vi "Sequence.vi"(8 "error in (no error)":errorcluster, 11 "Message Queues in":T73) -> (0 "error out":errorcluster)   [LabVIEW 2018, in "Sequencing Library.lvlib"]
uses:
  Sequencing Library.lvlib
  Main/Main Queue Cluster.ctl
  support/Message Queue/Message Cluster.ctl
  Drag and Drop/State Cluster.ctl
  Drag and Drop/Thumbnail Cluster.ctl
  Drag and Drop/Object Cluster.ctl
  <vilib>/Utility/miscctls.llb/LVRectTypeDef.ctl
  Drag and Drop/Object Type Enum.ctl
  <vilib>/Utility/miscctls.llb/LVPositionTypeDef.ctl
  Config Module/Controls/Main Config Cluster.ctl
  OPC/OPC Module Config.ctl
  Scale Module Folder/Measure Instrument/State Enum.ctl
  <vilib>/Utility/miscctls.llb/LVPoint32TypeDef.ctl
  OPC/OPC Settings.ctl
  OPC/Variable Data Cluster.ctl
  <vilib>/OPCUA/controls/NodeId.ctl
  <vilib>/OPCUA/controls/OPC UA StatusCode.ctl
  <vilib>/OPCUA/controls/Subscription ID.ctl
  <vilib>/OPCUA/controls/OPC UA Client Refnum.ctl
  <vilib>/OPCUA/controls/Subscription Data Change.ctl
  <vilib>/OPCUA/controls/Data Type.ctl
  OPC/OPC Tag Data.ctl
  Feed Module/Controls/Feed Module Config Cluster.ctl
  Feed Module/Controls/Feed Module Settings Cluster.ctl
  Ismatec ISM 831C/Controls/Ismatech ISM831C Settings Cluster.ctl
  Masterflex 7550-30/Controls/Settings Cluster.ctl
  Mettler Toledo/Controls/Settings Cluster.ctl
  Bronkhorst M13 Flow Meter/Settings Cluster.ctl
  Measure Instrument/PID 2 Parameters Cluster.ctl
  Measure Instrument/PID Input Enum.ctl
  Measure Instrument/PID 2 Output Enum.ctl
  Tacmina QI/Tacmina QI DAQ Setting.ctl
  KNF Pump/Settings Cluster plus SIMDOS.ctl
  ASIA Pump/Pump Settings.ctl
  VICI M50 Party Mode/Settings Cluster.ctl
  FLOM Pump/Settings Cluster.ctl
  SSI PR Class/SSI PR or LD Settings Cluster.ctl
  Masterflex 75211/Masterflex 75211 DAQ Setting.ctl
  SSI PR Class/SSI P40 Settings Cluster.ctl
  Ismatec 78001/Ismatec 4083.ctl
  Bronkhorst M14 Flow Meter/Settings Cluster.ctl
  TT Module/Controls/TT Module Config Cluster.ctl
  Tag VIs/Numeric Alarm Settings Cluster.ctl
  Acquisition/Hardware Configuration.ctl
  Acquisition/Task Cluster.ctl
  PT Module/Controls/PT Module Config Cluster.ctl
  Scale Module Folder/Feed Module/Controls/Scale Module Config Cluster.ctl
  Scale Module Folder/Feed Module/Controls/Scale Module Settings Cluster.ctl
  Pump Module Folder/Pump Module Config Cluster.ctl
  Pump Module Folder/Pump Module Settings Cluster.ctl
  LabJack Module/Controls/U3 Module Config Cluster.ctl
  Decoration Module/Decoration Module Config Cluster.ctl
  Flow Module Folder/Feed Module/Controls/Flow Module Config Cluster.ctl
  Flow Module Folder/Feed Module/Controls/Flow Module Settings Cluster.ctl
  TCU Module/TCU Module Folder/TCU Module Config Cluster.ctl
  TCU Module/TCU Module Folder/TCU Module Settings Cluster.ctl
  TCU Module/TCU Module Folder/Measure Instrument/Output Devices.ctl
  Huber TCU/Huber Settings.ctl
  Lauda Integral XT-150 TCU/Lauda Settings.ctl
  Julabo Type 1 TCU/Julabo Type 1 TCU Folder/Julabo FP-50 Settings.ctl
  Huber Unistat 410 TCU/Huber Unistat 410 RS485 Settings.ctl
  D-O Module Folder/Not Sure Where this is Used.ctl
  Squence Control.ctl
  D-O Module Folder/D-O Module Config Cluster.ctl
  D-O Module Folder/Valve Clusters.ctl
  D-O Module Folder/D-O Module Settings Cluster.ctl
  D-O Module Folder/D-O Device Settings Cluster.ctl
  VICI Electronic Actuator/VICI Electronic Actuator Settings.ctl
  Pressure Regulator Control Module/Pressure Regulator/Controls/4-20mA Module Config Cluster.ctl
  Pressure Regulator Control Module/Pressure Regulator/Controls/4-20mA Module Settings Cluster.ctl
  Pressure Transmitter/Pressure Transmitter Device Settings.ctl
  Pressure Reg Module/Pressure Regulator Device Settings.ctl
  Sonicator Module Folder/Feed Module/Controls/Sonicator Module Config Cluster.ctl
  Sonicator Module Folder/Feed Module/Controls/Sonicator Module Settings Cluster.ctl
  Sonic Systems P100/Sonic Systems P100 Settings.ctl
  Agitator Module Folder/Feed Module/Controls/Agitator Module Config Cluster.ctl
  Agitator Module Folder/Feed Module/Controls/Agitator Module Settings Cluster.ctl
  Squence Update Cluster.ctl
  support/Message Queue/Enqueue Message (Single).vi
  support/Message Queue/Message Queue.lvlib
  support/Command Log VIs/Command Logging.lvlib
  Drag and Drop/Drag and Drop.lvlib
  Config Module/Config Module.lvlib
  TT Module/TT Module.lvlib
  Feed Module/Feed Module.lvlib
  Ismatec ISM 831C/Ismatec ISM 831C.lvlib
  Masterflex 7550-30/Masterflex 7550-30.lvlib
  Mettler Toledo/Mettler Toledo.lvlib
  Bronkhorst M13 Flow Meter/Bronkhorst M13 Flow Meter.lvlib
  Tacmina QI/Tacmina QI.lvlib
  KNF Pump/KNF SIMDOS.lvlib
  ASIA Pump.lvlib
  DAQ/DAQ.lvlib
  PT Module/PT Module.lvlib
  Scale Module Folder/Scale Module.lvlib
  Pump Module Folder/Pump Module.lvlib
  LabJack Module/U3 Module.lvlib
  Flow Module Folder/Flow Module.lvlib
  TCU Module/TCU Module Folder/TCU Module.lvlib
  Huber TCU/Huber Ministat 230 TCU.lvlib
  Lauda Integral XT-150 TCU/Lauda TCU.lvlib
  Julabo Type 1 TCU/Julabo Type 1 TCU Folder/Julabo Type FP-50 TCU.lvlib
  VICI M50 Party Mode/VICI M6 M50 Party Mode.lvlib
  D-O Module Folder/D-O Module.lvlib
  Pressure Transmitter/Pressure Transmitter Library.lvlib
  Pressure Regulator Control Module/Pressure Regulator/4-20mA Module.lvlib
  Pressure Reg Module/Pressure Regulator Library.lvlib
  FLOM Pump/FLOM Pump.lvlib
  SSI PR Class/SSI PR or LD Pump.lvlib
  OPC/OPC UA.lvlib
  Scale Module Folder/Measure Instrument/Scale Module Engine.lvlib
  D-O Module Folder/DIO Valve/VICI Electronic Actuator.lvlib
  Masterflex 75211/Masterflex 75211.lvlib
  SSI PR Class/SSI P40 Pump.lvlib
  Huber Unistat 410 TCU/Huber Unistat 410 TCU.lvlib
  Ismatec 78001/Ismatec 4308.lvlib
  Bronkhorst M14 Flow Meter/Bronkhorst M14 Flow Meter.lvlib
  Sonicator Module Folder/Sonicator Module.lvlib
  Sonic Systems P100/Sonic Systems P100.lvlib
  Agitator Module Folder/Agitator Module.lvlib
panel:
  in  "Input 2":T1 {"Main Config"."PR Module Configs"."Settings"."PID 2 Parameters"."output range"."output low" format="%.2f"; "Main Config"."PR Module Configs"."Settings"."PID 2 Parameters"."output range"."output high" min=0.0 max=100.0 format="%.2f"; "Main Config"."PR Module Configs"."Settings"."PID 2 Parameters"."PID gains"."derivative time (Td, min)" format="%.3f"; "Main Config"."PR Module Configs"."Settings"."PID 2 Parameters"."PID gains"."integral time (Ti, min)" format="%.3f"; "Main Config"."PR Module Configs"."Settings"."PID 2 Parameters"."PID gains"."proportional gain (Kc)" format="%.3f"; "Main Config"."Steps"."Control" items=["Pump %", "Setpoint"]; "Main Config"."TCU Module Configs"."Settings"."Huber Unistat 410 Settings"."Address" min=0 max=99 format="%02.0f"; "Main Config"."TCU Module Configs"."Settings"."Julabo FP-50 Settings"."Pump Power" min=0 max=8 step=1; "Main Config"."TCU Module Configs"."Settings"."Lauda Settings"."Pump Power" min=0 max=8 step=1; "Main Config"."Flow Module Configs"."Settings"."Bronkhorst M14 Settings"."Smoothing Steps" min=1 step=1; "Main Config"."Flow Module Configs"."Settings"."Bronkhorst M13 Settings"."Smoothing Steps" min=1 step=1; "Main Config"."Pump Module Configs"."Settings"."Ismatech 3 Channel Settings"."Channel Number" min=0 max=3; "Main Config"."Pump Module Configs"."Settings"."Ismatech 3 Channel Settings"."Pump Number" min=1; "Main Config"."Pump Module Configs"."Settings"."ASIA Pump C"."channel" min=0 max=1 step=1; "Main Config"."Pump Module Configs"."Settings"."Masterflex"."Pump Number" min=1.0 max=20.0 step=1.0; "Main Config"."Pump Module Configs"."Settings"."Ismatech"."Pump Number" min=1.0 max=20.0 step=1.0; "Main Config"."Feed Module Configs"."Settings"."Bronkhorst M14 Settings"."Smoothing Steps" min=1 step=1; "Main Config"."Feed Module Configs"."Settings"."Ismatech 3 Channel Settings"."Channel Number" min=0 max=3; "Main Config"."Feed Module Configs"."Settings"."Ismatech 3 Channel Settings"."Pump Number" min=1; "Main Config"."Feed Module Configs"."Settings"."output range"."output low" min=0.0 max=100.0 format="%.2f"; "Main Config"."Feed Module Configs"."Settings"."output range"."output high" format="%.2f"; "Main Config"."Feed Module Configs"."Settings"."PID 2 Parameters"."PID gains"."derivative time (Td, min)" format="%.3f"; "Main Config"."Feed Module Configs"."Settings"."PID 2 Parameters"."PID gains"."integral time (Ti, min)" format="%.3f"; "Main Config"."Feed Module Configs"."Settings"."PID 2 Parameters"."PID gains"."proportional gain (Kc)" format="%.3f"; "Main Config"."Feed Module Configs"."Settings"."Bronkhorst M13 Flow Meter"."Smoothing Steps" min=1 step=1; "Main Config"."Feed Module Configs"."Settings"."ASIA Pump C"."channel" min=0 max=1 step=1; "Main Config"."Feed Module Configs"."Settings"."Ismatech"."Pump Number" min=1.0 max=20.0 step=1.0; "Main Config"."Feed Module Configs"."Settings"."Masterflex"."Pump Number" min=1.0 max=20.0 step=1.0}
  out "Metrics:Code Size":u32
  out "Metrics:Total Data Size":u32
  out "Application:All VIs In Memory":string[](array[string])
  out "error out 2":errorcluster
  out "Process Name":string
  out "Queue Name":string
  out "Loop Variable":u32
  out "Step":i32
  out "Done":bool
  out "Output":T1 {"Main Config"."PR Module Configs"."Settings"."PID 2 Parameters"."output range"."output low" format="%.2f"; "Main Config"."PR Module Configs"."Settings"."PID 2 Parameters"."output range"."output high" min=0.0 max=100.0 format="%.2f"; "Main Config"."PR Module Configs"."Settings"."PID 2 Parameters"."PID gains"."derivative time (Td, min)" format="%.3f"; "Main Config"."PR Module Configs"."Settings"."PID 2 Parameters"."PID gains"."integral time (Ti, min)" format="%.3f"; "Main Config"."PR Module Configs"."Settings"."PID 2 Parameters"."PID gains"."proportional gain (Kc)" format="%.3f"; "Main Config"."Steps"."Control" items=["Pump %", "Setpoint"]; "Main Config"."TCU Module Configs"."Settings"."Huber Unistat 410 Settings"."Address" min=0 max=99 format="%02.0f"; "Main Config"."TCU Module Configs"."Settings"."Julabo FP-50 Settings"."Pump Power" min=0 max=8 step=1; "Main Config"."TCU Module Configs"."Settings"."Lauda Settings"."Pump Power" min=0 max=8 step=1; "Main Config"."Flow Module Configs"."Settings"."Bronkhorst M14 Settings"."Smoothing Steps" min=1 step=1; "Main Config"."Flow Module Configs"."Settings"."Bronkhorst M13 Settings"."Smoothing Steps" min=1 step=1; "Main Config"."Pump Module Configs"."Settings"."Ismatech 3 Channel Settings"."Channel Number" min=0 max=3; "Main Config"."Pump Module Configs"."Settings"."Ismatech 3 Channel Settings"."Pump Number" min=1; "Main Config"."Pump Module Configs"."Settings"."ASIA Pump C"."channel" min=0 max=1 step=1; "Main Config"."Pump Module Configs"."Settings"."Masterflex"."Pump Number" min=1.0 max=20.0 step=1.0; "Main Config"."Pump Module Configs"."Settings"."Ismatech"."Pump Number" min=1.0 max=20.0 step=1.0; "Main Config"."Feed Module Configs"."Settings"."Bronkhorst M14 Settings"."Smoothing Steps" min=1 step=1; "Main Config"."Feed Module Configs"."Settings"."Ismatech 3 Channel Settings"."Channel Number" min=0 max=3; "Main Config"."Feed Module Configs"."Settings"."Ismatech 3 Channel Settings"."Pump Number" min=1; "Main Config"."Feed Module Configs"."Settings"."output range"."output low" min=0.0 max=100.0 format="%.2f"; "Main Config"."Feed Module Configs"."Settings"."output range"."output high" format="%.2f"; "Main Config"."Feed Module Configs"."Settings"."PID 2 Parameters"."PID gains"."derivative time (Td, min)" format="%.3f"; "Main Config"."Feed Module Configs"."Settings"."PID 2 Parameters"."PID gains"."integral time (Ti, min)" format="%.3f"; "Main Config"."Feed Module Configs"."Settings"."PID 2 Parameters"."PID gains"."proportional gain (Kc)" format="%.3f"; "Main Config"."Feed Module Configs"."Settings"."Bronkhorst M13 Flow Meter"."Smoothing Steps" min=1 step=1; "Main Config"."Feed Module Configs"."Settings"."ASIA Pump C"."channel" min=0 max=1 step=1; "Main Config"."Feed Module Configs"."Settings"."Ismatech"."Pump Number" min=1.0 max=20.0 step=1.0; "Main Config"."Feed Module Configs"."Settings"."Masterflex"."Pump Number" min=1.0 max=20.0 step=1.0}
  out "Intruction Cluster":T58 {"Control" items=["Setpoint", "Pump %"]}
  out "Paused":bool
  out "Stop":bool
  in  "Input":T1 {"Main Config"."PR Module Configs"."Settings"."PID 2 Parameters"."output range"."output low" format="%.2f"; "Main Config"."PR Module Configs"."Settings"."PID 2 Parameters"."output range"."output high" min=0.0 max=100.0 format="%.2f"; "Main Config"."PR Module Configs"."Settings"."PID 2 Parameters"."PID gains"."derivative time (Td, min)" format="%.3f"; "Main Config"."PR Module Configs"."Settings"."PID 2 Parameters"."PID gains"."integral time (Ti, min)" format="%.3f"; "Main Config"."PR Module Configs"."Settings"."PID 2 Parameters"."PID gains"."proportional gain (Kc)" format="%.3f"; "Main Config"."Steps"."Control" items=["Pump %", "Setpoint"]; "Main Config"."TCU Module Configs"."Settings"."Huber Unistat 410 Settings"."Address" min=0 max=99 format="%02.0f"; "Main Config"."TCU Module Configs"."Settings"."Julabo FP-50 Settings"."Pump Power" min=0 max=8 step=1; "Main Config"."TCU Module Configs"."Settings"."Lauda Settings"."Pump Power" min=0 max=8 step=1; "Main Config"."Flow Module Configs"."Settings"."Bronkhorst M14 Settings"."Smoothing Steps" min=1 step=1; "Main Config"."Flow Module Configs"."Settings"."Bronkhorst M13 Settings"."Smoothing Steps" min=1 step=1; "Main Config"."Pump Module Configs"."Settings"."Ismatech 3 Channel Settings"."Channel Number" min=0 max=3; "Main Config"."Pump Module Configs"."Settings"."Ismatech 3 Channel Settings"."Pump Number" min=1; "Main Config"."Pump Module Configs"."Settings"."ASIA Pump C"."channel" min=0 max=1 step=1; "Main Config"."Pump Module Configs"."Settings"."Masterflex"."Pump Number" min=1.0 max=20.0 step=1.0; "Main Config"."Pump Module Configs"."Settings"."Ismatech"."Pump Number" min=1.0 max=20.0 step=1.0; "Main Config"."Feed Module Configs"."Settings"."Bronkhorst M14 Settings"."Smoothing Steps" min=1 step=1; "Main Config"."Feed Module Configs"."Settings"."Ismatech 3 Channel Settings"."Channel Number" min=0 max=3; "Main Config"."Feed Module Configs"."Settings"."Ismatech 3 Channel Settings"."Pump Number" min=1; "Main Config"."Feed Module Configs"."Settings"."output range"."output low" min=0.0 max=100.0 format="%.2f"; "Main Config"."Feed Module Configs"."Settings"."output range"."output high" format="%.2f"; "Main Config"."Feed Module Configs"."Settings"."PID 2 Parameters"."PID gains"."derivative time (Td, min)" format="%.3f"; "Main Config"."Feed Module Configs"."Settings"."PID 2 Parameters"."PID gains"."integral time (Ti, min)" format="%.3f"; "Main Config"."Feed Module Configs"."Settings"."PID 2 Parameters"."PID gains"."proportional gain (Kc)" format="%.3f"; "Main Config"."Feed Module Configs"."Settings"."Bronkhorst M13 Flow Meter"."Smoothing Steps" min=1 step=1; "Main Config"."Feed Module Configs"."Settings"."ASIA Pump C"."channel" min=0 max=1 step=1; "Main Config"."Feed Module Configs"."Settings"."Ismatech"."Pump Number" min=1.0 max=20.0 step=1.0; "Main Config"."Feed Module Configs"."Settings"."Masterflex"."Pump Number" min=1.0 max=20.0 step=1.0}
  # "Agitator Settings"
  # "Sonicator Settings"
  # "Instrument Settings"
  # "Instrument Settings"
  # "Output Instruments"
  # "Flow Meter Settings"
  # "Output Instruments"
  # "Scale Settings"
  # "Output Instruments"
  # "Input Instruments"
  # "Agitator Settings"
  # "Sonicator Settings"
  # "Instrument Settings"
  # "Instrument Settings"
  # "Output Instruments"
  # "Flow Meter Settings"
  # "Output Instruments"
  # "Scale Settings"
  # "Output Instruments"
  # "Input Instruments"
  # "Agitator Settings"
  # "Sonicator Settings"
  # "Instrument Settings"
  # "Instrument Settings"
  # "Output Instruments"
  # "Flow Meter Settings"
  # "Output Instruments"
  # "Scale Settings"
  # "Output Instruments"
  # "Input Instruments"
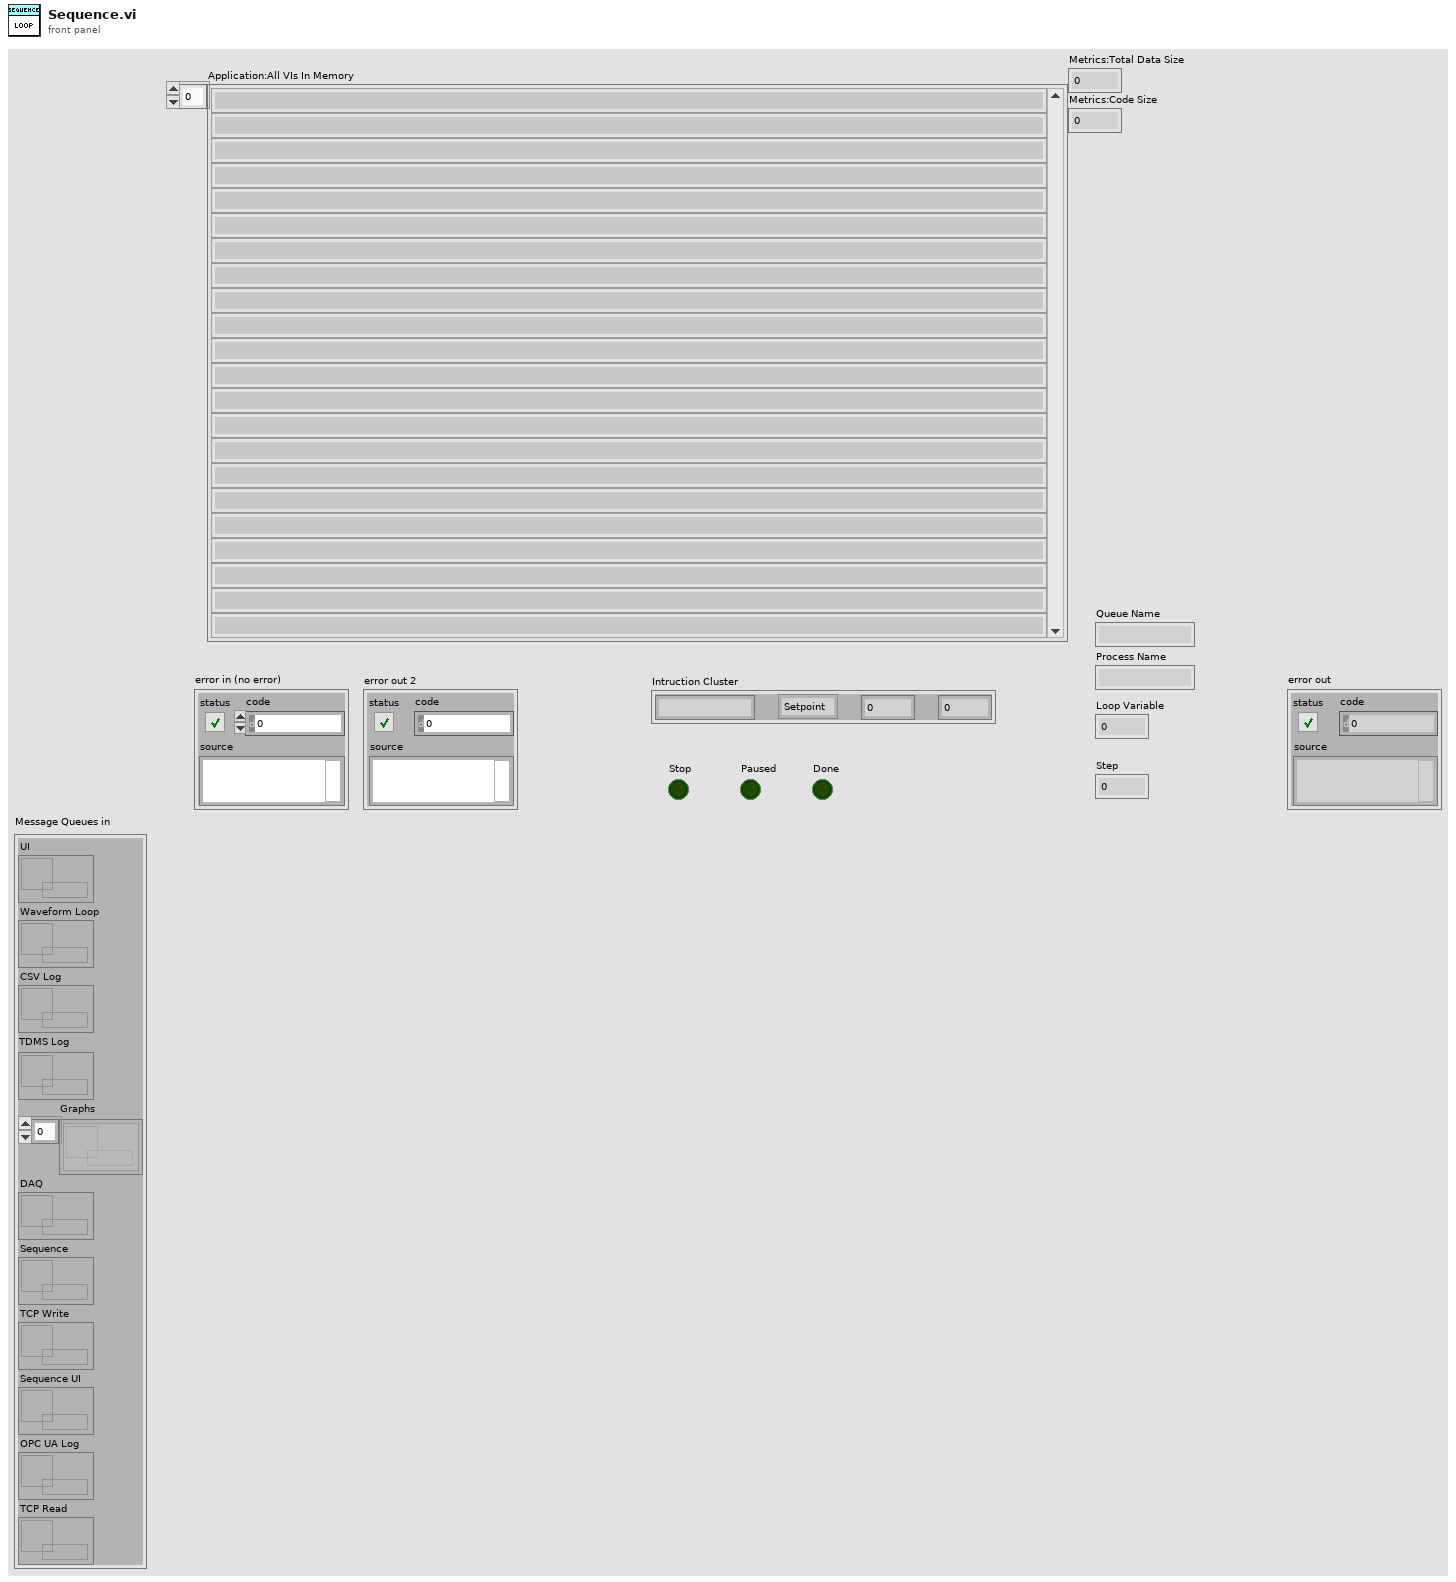
[diagram p1: front panel]
types:
  T1 = typedef "Drag and Drop.lvlib/State Cluster.ctl" = cluster{"VI refs":refnum<vi>[], "Queues":refnum<queue>[], "[Thumbnails]":T2[], "Drag Object Idx":i32, "[Objects]":T3[], "Active Object":i32, "Drop Offset":T6, "Process Name":string, "Main Config":T7, "Campaign Filepath":path, "Config Changed?":bool}
  T2 = typedef "Thumbnail Cluster.ctl" = cluster{"Path":path, "Rectangle":cluster{"left":i16, "top":i16, "right":i16, "bottom":i16}}
  T3 = typedef "Object Cluster.ctl" = cluster{"BMP Path":path, "Anchor Position":cluster{"X":i32, "Y":i32}, "Hot Spot":T4, "Type":T5, "Parameters":variant}
  T4 = typedef "LVRectTypeDef.ctl" = cluster{"Left":i16, "Top":i16, "Right":i16, "Bottom":i16}
  T5 = typedef "Object Type Enum.ctl" = enum16{"Icon", "Line", "Text", "Feed Module"}
  T6 = typedef "LVPositionTypeDef.ctl" = cluster{"Left":i32, "Top":i32}
  T7 = typedef "Config Module.lvlib/Main Config Cluster.ctl" = cluster{"Notebook":string, "OPC Module Configs":T8[], "Feed Module Configs":T18[], "Log File Path":path, "TT Module Configs":T37[], "DAQ Config":T39, "PT Module Configs":T41[], "Scale Module Configs":T42[], "Pump Module Configs":T44[], "U3 Module Configs":T46[], "Decoration Module Configs":T47[], "Flow Module Configs":T48[], "TCU Module Configs":T50[], "Steps":T57, "Abort":bool, "DO Module Configs":T59[], "PR Module Configs":T64[], "SC Module Configs":T68[], "AM Module Configs":T71[], "Cycle Period":dbl}
  T8 = typedef "OPC UA.lvlib/OPC Module Config.ctl" = cluster{"State":T9, "GUID":string, "Drop Coords":T10, "Configuration":T11, "First Iteration":bool, "Data":cluster{"Object Name":string, "Variable Array":T12[]}[], "Process Name":string, "Load Count":i32, "Log Started":bool, "subscription ID out":T15, "OPC UA client refnum out":T16, "Event Registration Refnum":refnum<event-registration>, "Start Time":timestamp, "Current Time":timestamp, "Tag Data":T17[]}
  T9 = typedef "Scale Module.lvlib/Scale Module Engine.lvlib/State Enum.ctl" = enum16{"Measuring", "Idle"}
  T10 = typedef "LVPoint32TypeDef.ctl" = cluster{"Horizontal":i32, "Vertical":i32}
  T11 = typedef "OPC UA.lvlib/OPC Settings.ctl" = cluster{"Cycle Period":dbl, "server endpoint URL":string, "security policy":cluster{"message mode":enum16{"None", "Sign", "Sign and Encrypt"}, "security":enum16{"Basic256", "Basic128Rsa15"}}, "Trust Any Server":bool}
  T12 = typedef "OPC UA.lvlib/Variable Data Cluster.ctl" = cluster{"node ID":T13, "browse name":string, "status":T14, "timestamp":timestamp, "value ":variant}
  T13 = typedef "NodeId.ctl" = string
  T14 = typedef "OPC UA StatusCode.ctl" = u32
  T15 = typedef "Subscription ID.ctl" = u32
  T16 = typedef "OPC UA Client Refnum.ctl" = refnum<k21>
  T17 = typedef "OPC UA.lvlib/OPC Tag Data.ctl" = cluster{"Include this Device":bool, "Device Name":string, "OPC Tag Data":cluster{"Tag":string, "Value":variant, "Time Stamp":timestamp}[]}
  T18 = typedef "Feed Module.lvlib/Feed Module Config Cluster.ctl" = cluster{"GUID":string, "Drop Coords":T10, "Process Name":string, "Queue Name":string, "Settings":T19, "Settings Load Count":i32, "OP Load Count":i32}
  T19 = typedef "Feed Module.lvlib/Feed Module Settings Cluster.ctl" = cluster{"Cycle Period":dbl, "Ismatech":T20, "Masterflex":T21, "Mettler":T22, "Bronkhorst M13 Flow Meter":T23, "PID 2 Parameters":T24, "Manual Entry":dbl, "Auto?":bool, "output range":cluster{"output high":dbl, "output low":dbl}, "Tacmina Settings":T27, "KNF SIMDOS Settings":T28, "ASIA Pump C":T29, "VICI Settings":T30, "FLOM Settings":T31, "SSI PR/LD Settings":T32, "Masterflex 75211 Settings":T33, "SSI P40 Settings":T34, "Ismatech 3 Channel Settings":T35, "Bronkhorst M14 Settings":T36}
  T20 = typedef "Ismatec ISM 831C.lvlib/Ismatech ISM831C Settings Cluster.ctl" = cluster{"VISA resource name":refnum<visa-resource-name>, "Simulated?":bool, "Pump Number":dbl, "Reverse?":bool}
  T21 = typedef "Masterflex 7550-30.lvlib/Settings Cluster.ctl" = cluster{"VISA resource name":refnum<visa-resource-name>, "Simulated?":bool, "Pump Number":dbl, "Reverse?":bool}
  T22 = typedef "Mettler Toledo.lvlib/Settings Cluster.ctl" = cluster{"VISA resource name":refnum<visa-resource-name>, "Simulated?":bool}
  T23 = typedef "Bronkhorst M13 Flow Meter.lvlib/Settings Cluster.ctl" = cluster{"VISA resource name":refnum<visa-resource-name>, "Simulated?":bool, "Smoothing Steps":i32}
  T24 = typedef "PID 2 Parameters Cluster.ctl" = cluster{"Input Device":T25, "Output Device":T26, "Setpoint":dbl, "PID gains":cluster{"proportional gain (Kc)":dbl, "integral time (Ti, min)":dbl, "derivative time (Td, min)":dbl}}
  T25 = typedef "PID Input Enum.ctl" = enum16{"Default", "Bronkhorst M13", "Bronkhorst M14", "Scale Rate of Change"}
  T26 = typedef "PID 2 Output Enum.ctl" = enum16{"Default", "Ismatec ISM 4308", "Ismatec ISM 831C", "Masterflex 7550-30", "VICI", "Tacmina QI", "KNF SIMDOS", "ASIA Type C", "FLOM UI-22-11", "SSI PR/LD", "SSI P40", "Masterflex 75211-70"}
  T27 = typedef "Tacmina QI.lvlib/Tacmina QI DAQ Setting.ctl" = cluster{"Analog DAQ Task":refnum<k21>, "Digital DAQ Task":refnum<k21>}
  T28 = typedef "KNF SIMDOS.lvlib/Settings Cluster plus SIMDOS.ctl" = cluster{"VISA resource name":refnum<visa-resource-name>, "Simulated?":bool}
  T29 = typedef "ASIA Pump.lvlib/Pump Settings.ctl" = cluster{"ASIA Pump #":i32, "channel":i32, "Simulated":bool}
  T30 = typedef "VICI M6 M50 Party Mode.lvlib/Settings Cluster.ctl" = cluster{"VISA resource name":refnum<visa-resource-name>, "Simulated?":bool, "Pump Letter":string, "Reverse?":bool}
  T31 = typedef "FLOM Pump.lvlib/Settings Cluster.ctl" = cluster{"VISA resource name":refnum<visa-resource-name>, "Simulated?":bool, "Pump Number":dbl}
  T32 = typedef "SSI PR or LD Pump.lvlib/SSI PR or LD Settings Cluster.ctl" = cluster{"VISA resource name":refnum<visa-resource-name>, "Simulated?":bool}
  T33 = typedef "Masterflex 75211.lvlib/Masterflex 75211 DAQ Setting.ctl" = cluster{"Analog DAQ Task":refnum<k21>, "Digital DAQ Task":refnum<k21>}
  T34 = typedef "SSI P40 Pump.lvlib/SSI P40 Settings Cluster.ctl" = cluster{"VISA resource name":refnum<visa-resource-name>, "Simulated?":bool}
  T35 = typedef "Ismatec 4308.lvlib/Ismatec 4083.ctl" = cluster{"VISA resource name":refnum<visa-resource-name>, "Pump Number":i16, "Channel Number":i16, "Simulated?":bool, "Reverse?":bool}
  T36 = typedef "Bronkhorst M14 Flow Meter.lvlib/Settings Cluster.ctl" = cluster{"VISA resource name":refnum<visa-resource-name>, "Simulated?":bool, "Smoothing Steps":i32}
  T37 = typedef "TT Module.lvlib/TT Module Config Cluster.ctl" = cluster{"GUID":string, "Drop Coords":T10, "Input Channel Tag Name ":string, "Process Name":string, "Queue Name":string, "Input Channel Numeric Alarm Settings":T38[]}
  T38 = typedef "Numeric Alarm Settings Cluster.ctl" = cluster{"enable? (F)":bool, "name":string, "alarm type":enum16{"HI_HI", "HI", "LO", "LO_LO"}, "level/change":dbl, "deadband/time":dbl, "alarm delay":dbl, "priority":u32, "ack type":enum16{"Auto", "User", "None", "Each Occurrence"}, "area":string, "description":string, "log? (T)":bool}
  T39 = typedef "DAQ.lvlib/Hardware Configuration.ctl" = cluster{"Tasks":T40[]}
  T40 = typedef "Task Cluster.ctl" = cluster{"DAQmx Task":refnum<k21>, "Read-Write Radio":enum32{"Read", "Write"}}
  T41 = typedef "PT Module.lvlib/PT Module Config Cluster.ctl" = cluster{"GUID":string, "Drop Coords":T10, "Input Channel Tag Name ":string, "Process Name":string, "Queue Name":string, "Input Channel Numeric Alarm Settings":T38[]}
  T42 = typedef "Scale Module.lvlib/Scale Module Config Cluster.ctl" = cluster{"GUID":string, "Drop Coords":T10, "Process Name":string, "Queue Name":string, "Settings":T43, "Load Count":i32}
  T43 = typedef "Scale Module.lvlib/Scale Module Settings Cluster.ctl" = cluster{"Cycle Period":dbl, "Mettler":T22, "Scale Type":string}
  T44 = typedef "Pump Module.lvlib/Pump Module Config Cluster.ctl" = cluster{"GUID":string, "Drop Coords":T10, "Process Name":string, "Queue Name":string, "Settings":T45, "Load Count":i32}
  T45 = typedef "Pump Module.lvlib/Pump Module Settings Cluster.ctl" = cluster{"Cycle Period":dbl, "Manual Entry":dbl, "Output Device":T26, "Ismatech":T20, "Ismatech 3 Channel Settings":T35, "Masterflex":T21, "VICI Settings":T30, "Tacmina Settings":T27, "KNF SIMDOS Settings":T28, "ASIA Pump C":T29, "FLOM Settings":T31, "SSI PR/LD Settings":T32, "SSI P40 Settings":T32, "Masterflex 75211 Settings":T33, "Pump Calibration File":path, "Calibration Slope":dbl, "Calibration Y Intercept":dbl, "Pump Cal Enum":u16}
  T46 = typedef "U3 Module.lvlib/U3 Module Config Cluster.ctl" = cluster{"GUID":string, "Drop Coords":T10, "AI Channel Number":enum16{"Default", "AI0", "AI1", "AI2", "AI3", "AI4", "AI5", "AI6", "AI7"}, "Process Name":string, "Queue Name":string, "Input Channel Numeric Alarm Settings":T38[]}
  T47 = typedef "Decoration Module Config Cluster.ctl" = cluster{"GUID":string, "Drop Coords":T10, "Decoration Filepath":path}
  T48 = typedef "Flow Module.lvlib/Flow Module Config Cluster.ctl" = cluster{"GUID":string, "Drop Coords":T10, "Process Name":string, "Queue Name":string, "Settings":T49, "Load Count":i32}
  T49 = typedef "Flow Module.lvlib/Flow Module Settings Cluster.ctl" = cluster{"Cycle Period":dbl, "Flow Meter Type":string, "Bronkhorst M13 Settings":T23, "Bronkhorst M14 Settings":T36}
  T50 = typedef "TCU Module.lvlib/TCU Module Config Cluster.ctl" = cluster{"GUID":string, "Drop Coords":T10, "Process Name":string, "Queue Name":string, "Settings":T51, "Load Count":i32, "Power Level Changed":bool}
  T51 = typedef "TCU Module.lvlib/TCU Module Settings Cluster.ctl" = cluster{"Cycle Period":dbl, "Setpoint Entry":dbl, "Output Device":T52, "Huber Ministat 230 Settings":T53, "Lauda Settings":T54, "Julabo FP-50 Settings":T55, "Internal Control?":bool, "Huber Unistat 410 Settings":T56}
  T52 = typedef "Output Devices.ctl" = enum16{"Default", "Huber Ministat 230", "Huber Unistat 410", "Lauda XT-150", "Julabo FP-50"}
  T53 = typedef "Huber Ministat 230 TCU.lvlib/Huber Settings.ctl" = cluster{"VISA resource name":refnum<visa-resource-name>, "Simulated?":bool}
  T54 = typedef "Lauda TCU.lvlib/Lauda Settings.ctl" = cluster{"VISA resource name":refnum<visa-resource-name>, "Simulated?":bool, "Pump Power":i32}
  T55 = typedef "Julabo Type FP-50 TCU.lvlib/Julabo FP-50 Settings.ctl" = cluster{"VISA resource name":refnum<visa-resource-name>, "Simulated?":bool, "Pump Power":i32}
  T56 = typedef "Huber Unistat 410 TCU.lvlib/Huber Unistat 410 RS485 Settings.ctl" = cluster{"VISA resource name":refnum<visa-resource-name>, "Address":i8, "Simulated?":bool}
  T57 = typedef "Not Sure Where this is Used.ctl" = T58[]
  T58 = typedef "Sequencing Library.lvlib/Squence Control.ctl" = cluster{"Module":string, "Control":u16, "Value":dbl, "Wait (sec)":dbl}
  T59 = typedef "D-O Module.lvlib/D-O Module Config Cluster.ctl" = cluster{"GUID":string, "Drop Coords":T10, "Process Name":string, "Queue Name":string, "Settings":T60, "Load Count":i32}
  T60 = typedef "D-O Module.lvlib/Valve Clusters.ctl" = cluster{"Valve Settings":T61, "Valve Type":enum16{"Default", "Digital Output Valve", "VICI Electronic Actuator"}, "Time On (Sec)":dbl, "Time Off (Sec)":dbl, "Run?":bool}
  T61 = typedef "D-O Module.lvlib/D-O Module Settings Cluster.ctl" = cluster{"D-O Settings":T62, "VICI Electronic Actuator":T63}
  T62 = typedef "D-O Module.lvlib/D-O Device Settings Cluster.ctl" = cluster{"DAQmx Task Name":refnum<k21>, "Output Channel":u16, "Output Channel Names":string[]}
  T63 = typedef "VICI Electronic Actuator.lvlib/VICI Electronic Actuator Settings.ctl" = cluster{"VISA resource name":refnum<visa-resource-name>, "Mode":enum16{"Two Positions With Stops", "Two Positions Without Stops", "Mutiposition"}, "Simulated":bool}
  T64 = typedef "4-20mA Module.lvlib/4-20mA Module Config Cluster.ctl" = cluster{"GUID":string, "Drop Coords":T10, "Process Name":string, "Queue Name":string, "Settings":T65, "Settings Load Count":i32}
  T65 = typedef "4-20mA Module.lvlib/4-20mA Module Settings Cluster.ctl" = cluster{"Cycle Period":dbl, "PID 2 Parameters":cluster{"Input Device":enum16{"Default", "4-20mA"}, "Output Device":enum16{"Default", "Equilibar Pressure Reg", "Flow Regulator"}, "Setpoint":dbl, "PID gains":cluster{"proportional gain (Kc)":dbl, "integral time (Ti, min)":dbl, "derivative time (Td, min)":dbl}, "output range":cluster{"output low":dbl, "output high":dbl}}, "Manual Entry":dbl, "Auto?":bool, "4-20mA Input Settings":T66, "4-20mA Out Settings":T67, "Input Channel Tag Name ":string}
  T66 = typedef "Pressure Transmitter Library.lvlib/Pressure Transmitter Device Settings.ctl" = cluster{"Input Channel ":u16}
  T67 = typedef "Pressure Regulator Library.lvlib/Pressure Regulator Device Settings.ctl" = cluster{"Output DAQ Task":refnum<k21>}
  T68 = typedef "Sonicator Module.lvlib/Sonicator Module Config Cluster.ctl" = cluster{"GUID":string, "Drop Coords":T10, "Process Name":string, "Queue Name":string, "Settings":T69, "Load Count":i32}
  T69 = typedef "Sonicator Module.lvlib/Sonicator Module Settings Cluster.ctl" = cluster{"Cycle Period":dbl, "Sonicator Type":string, "SS P100 Settings":T70, "Setpoint (µm)":dbl, "Cutoff (W)":dbl}
  T70 = typedef "Sonic Systems P100.lvlib/Sonic Systems P100 Settings.ctl" = cluster{"VISA resource name":refnum<visa-resource-name>, "Simulated?":bool}
  T71 = typedef "Agitator Module.lvlib/Agitator Module Config Cluster.ctl" = cluster{"GUID":string, "Drop Coords":T10, "Process Name":string, "Queue Name":string, "Settings":T72, "Load Count":i32}
  T72 = typedef "Agitator Module.lvlib/Agitator Module Settings Cluster.ctl" = cluster{"Cycle Period":dbl, "Agitator Type":string, "Setpoint (µm)":dbl}
  T73 = typedef "Main Queue Cluster.ctl" = cluster{"UI":refnum<queue>, "Waveform Loop":refnum<queue>, "CSV Log":refnum<queue>, "TDMS Log":refnum<queue>, "Graphs":refnum<queue>[], "DAQ":refnum<queue>, "Sequence":refnum<queue>, "TCP Write":refnum<queue>, "Sequence UI":refnum<queue>, "OPC UA Log":refnum<queue>, "TCP Read":refnum<queue>}
  T74 = typedef "Sequencing Library.lvlib/Squence Update Cluster.ctl" = cluster{"Auto?":bool, "Manual Entry":dbl, "Setpoint":dbl}
  T75 = enum16{"open", "replace", "create", "open or create", "replace or create", "replace or create with confirmation"}
  T76 = typedef "Support Library.lvlib/Message Queue.lvlib/Message Cluster.ctl" = cluster{"Message":string, "Message Data":variant}
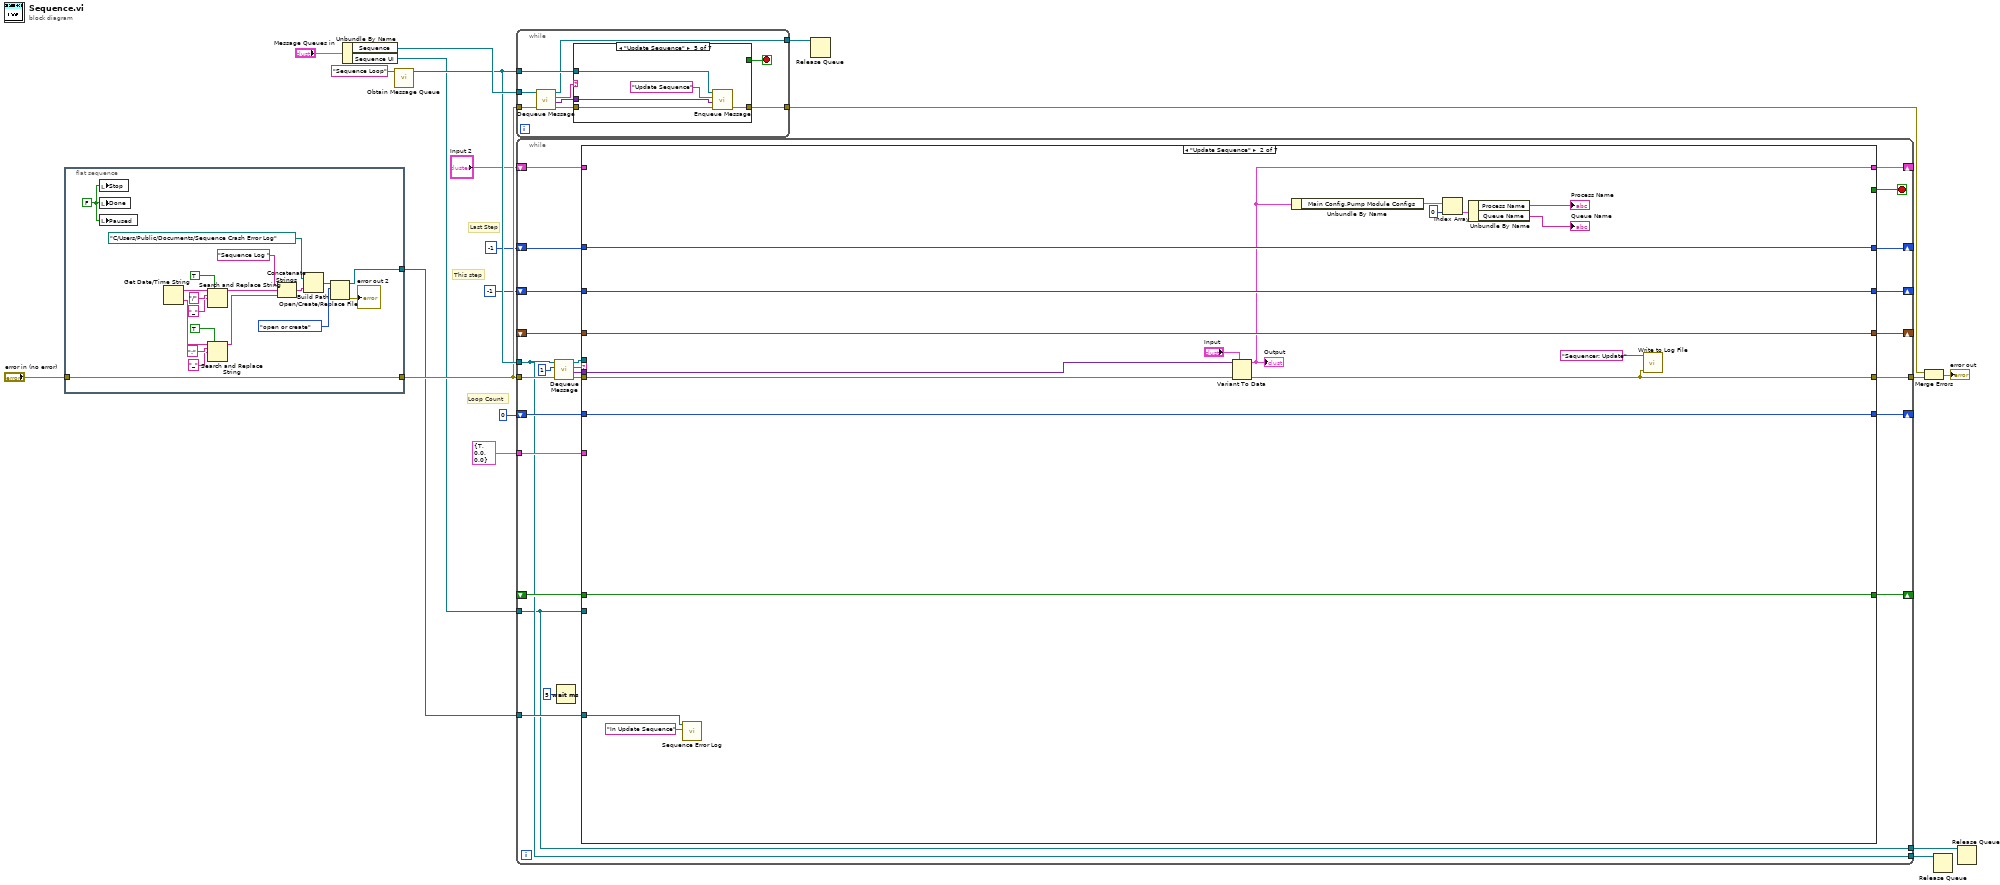
[diagram p0: block diagram]
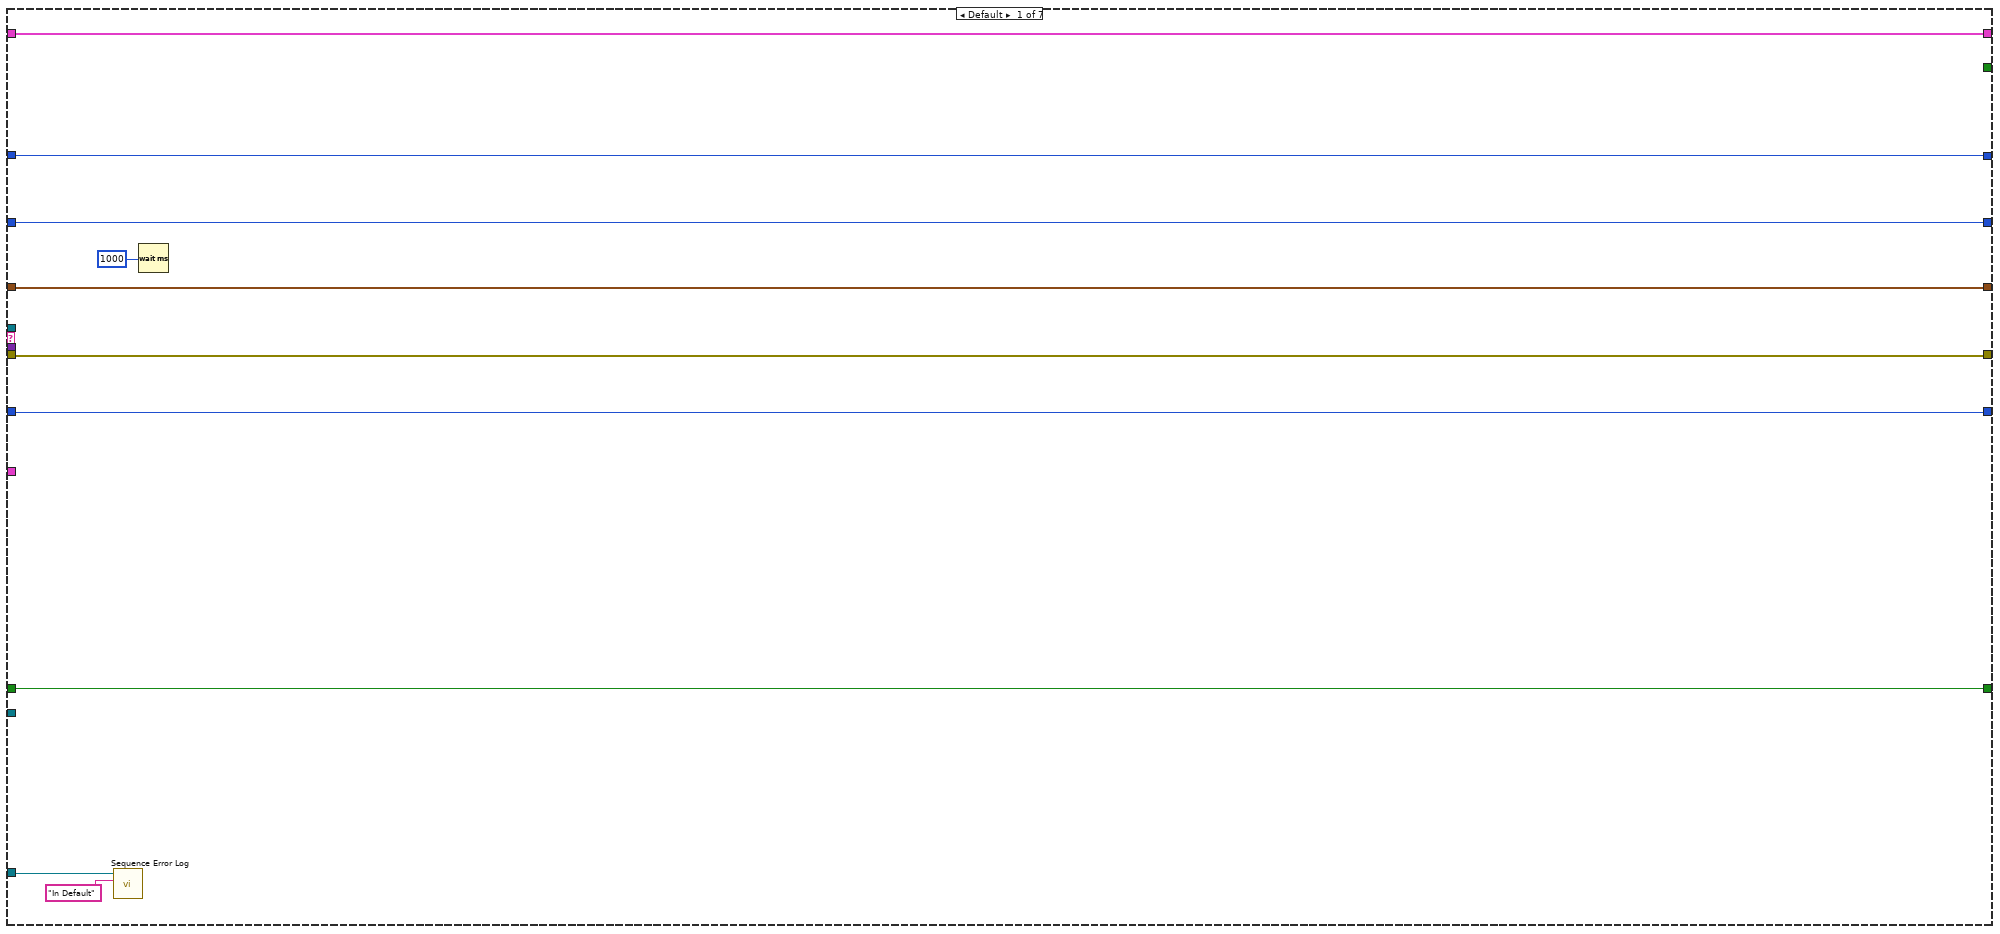
[diagram p2: hidden frame]
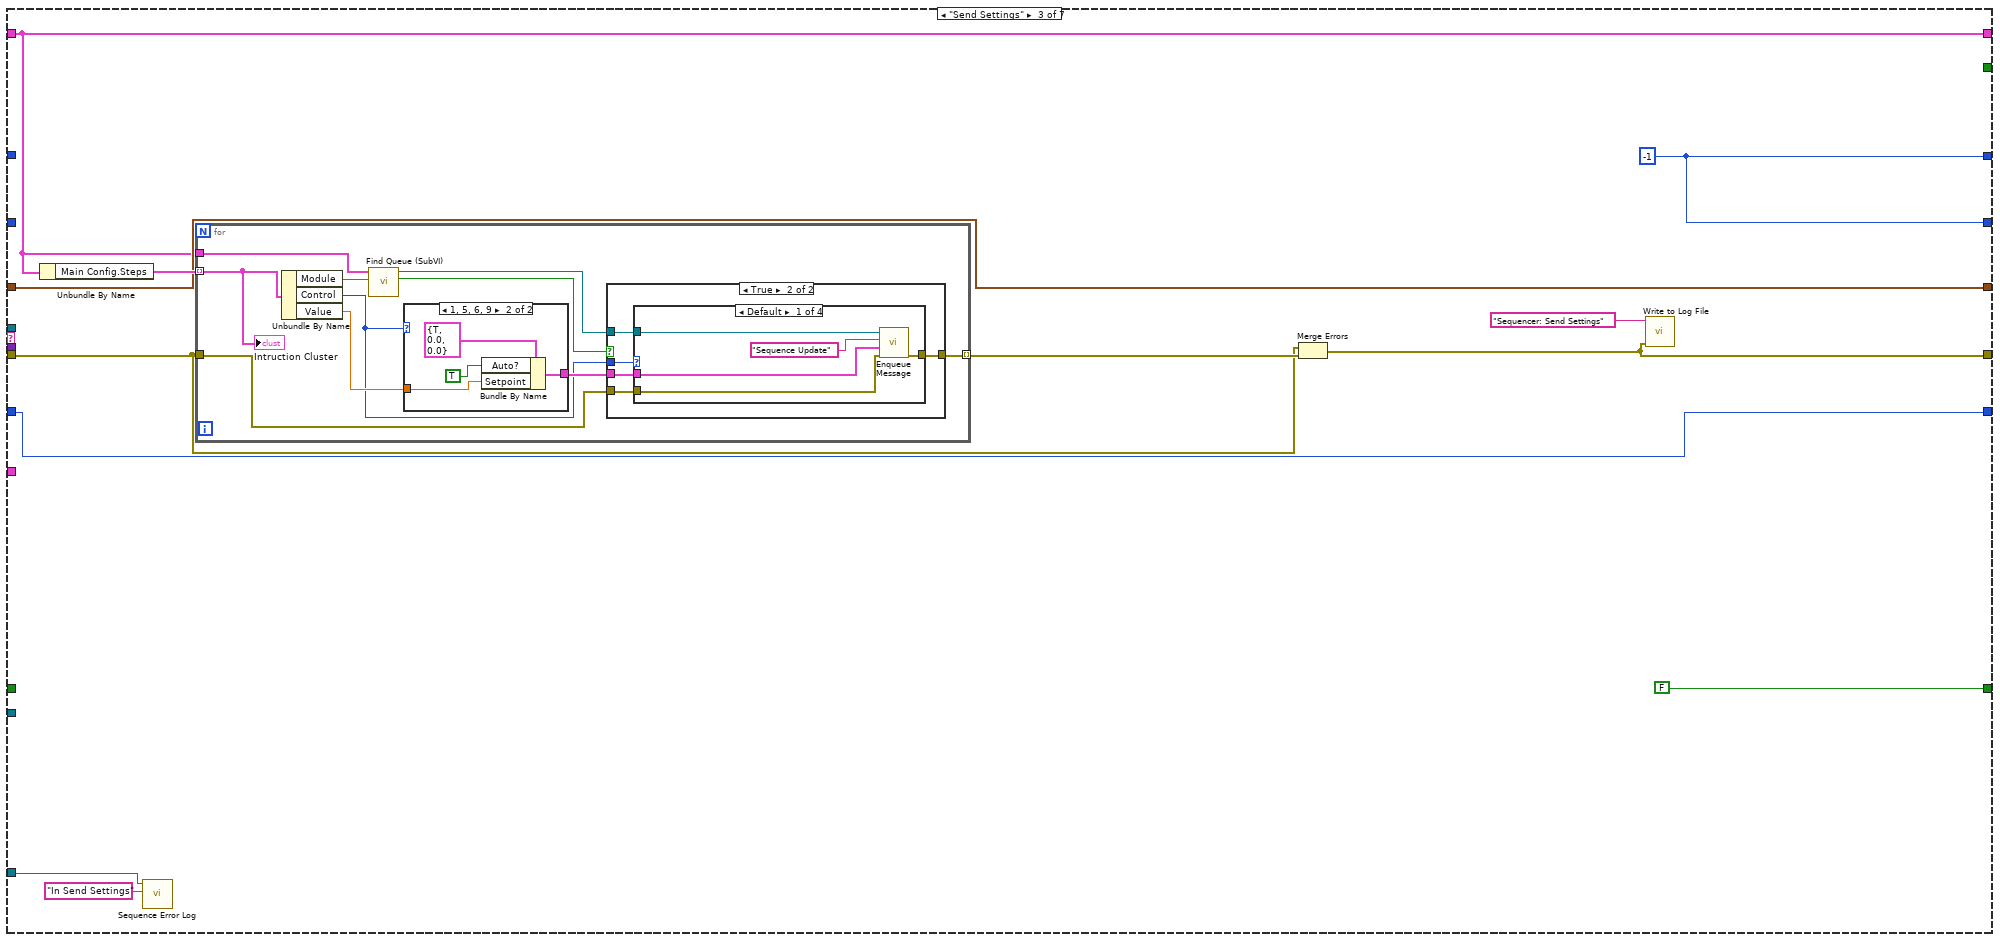
[diagram p3: hidden frame]
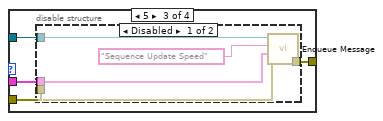
[diagram p6: hidden frame]
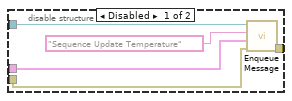
[diagram p9: hidden frame]
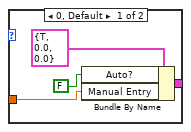
[diagram p10: hidden frame]
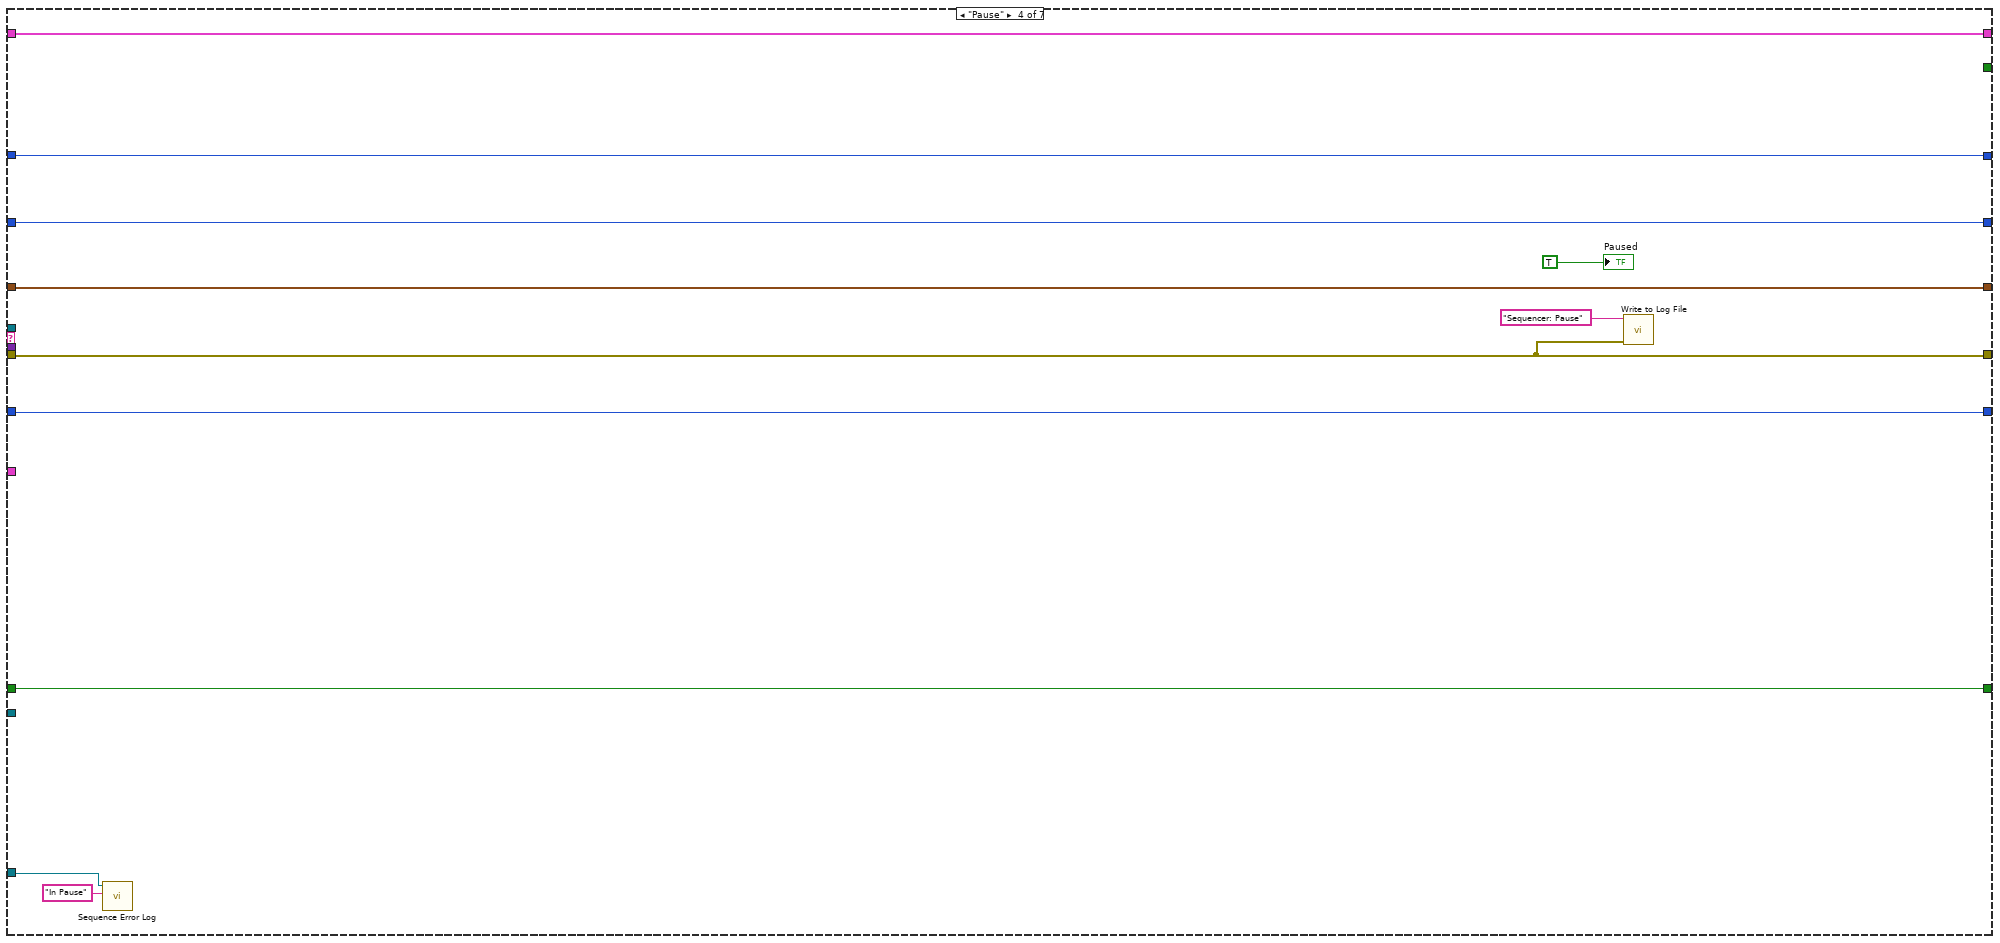
[diagram p11: hidden frame]
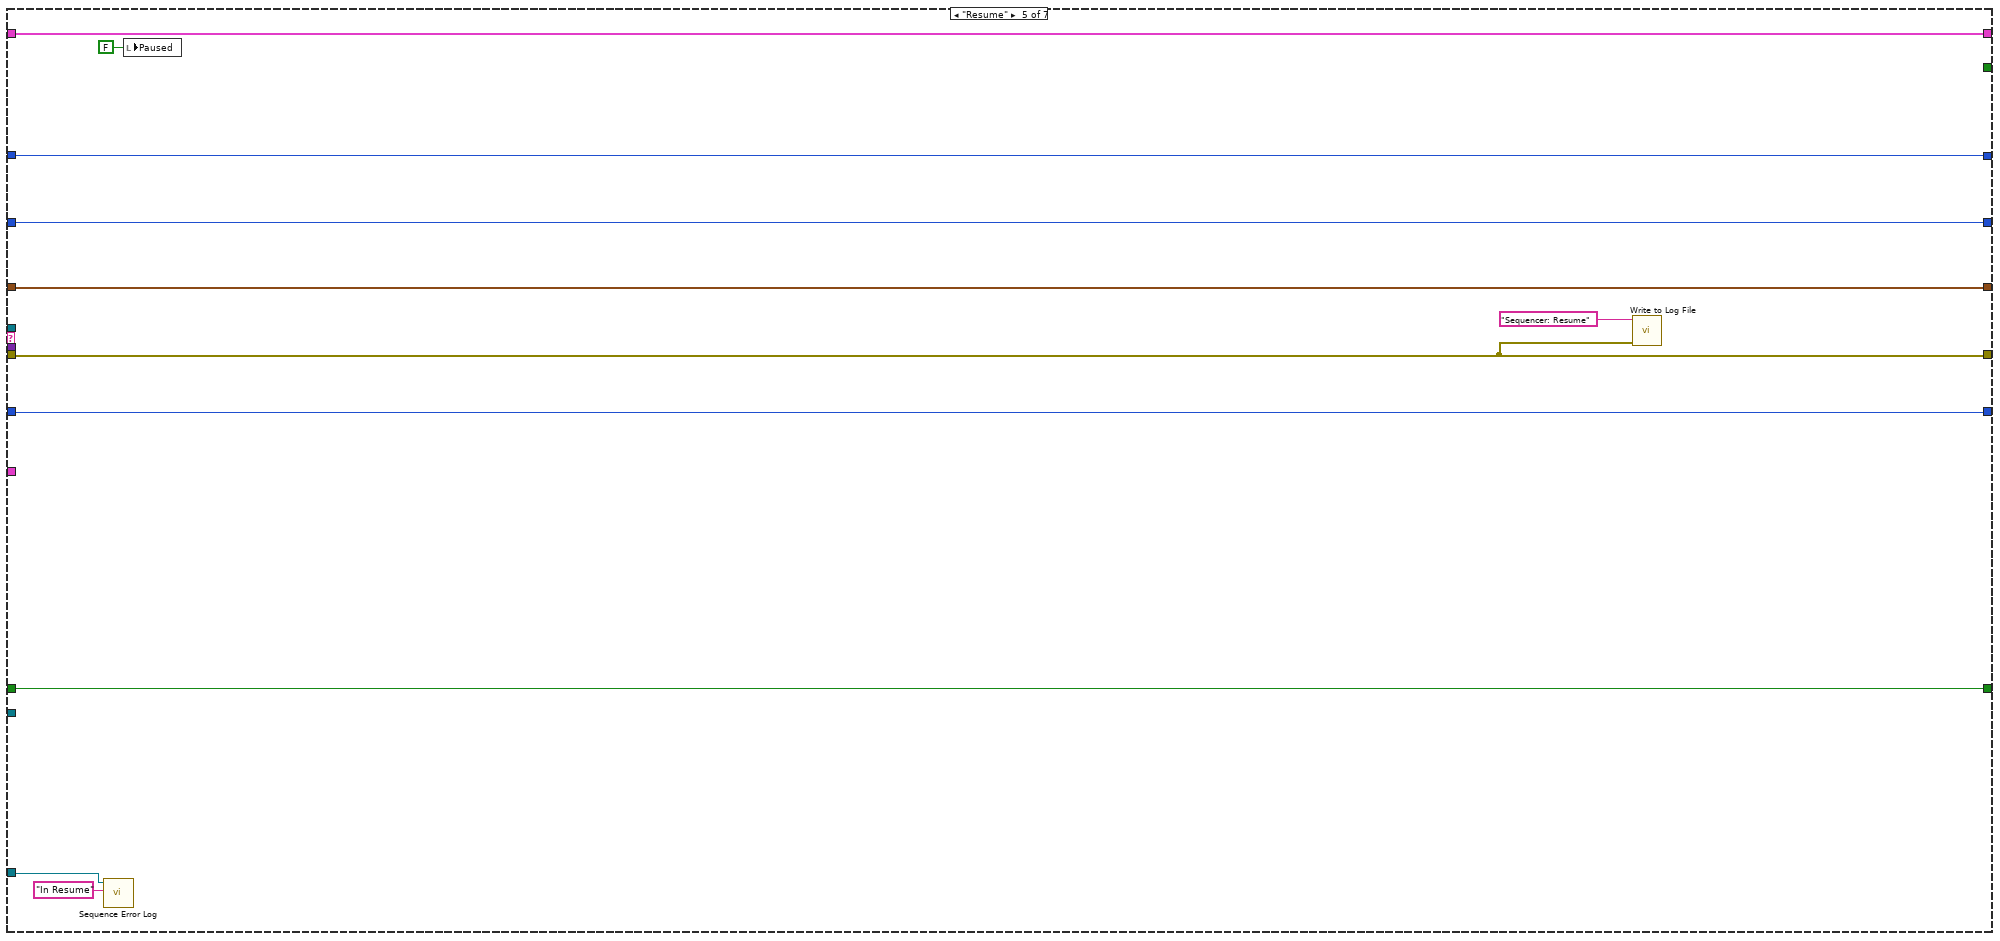
[diagram p12: hidden frame]
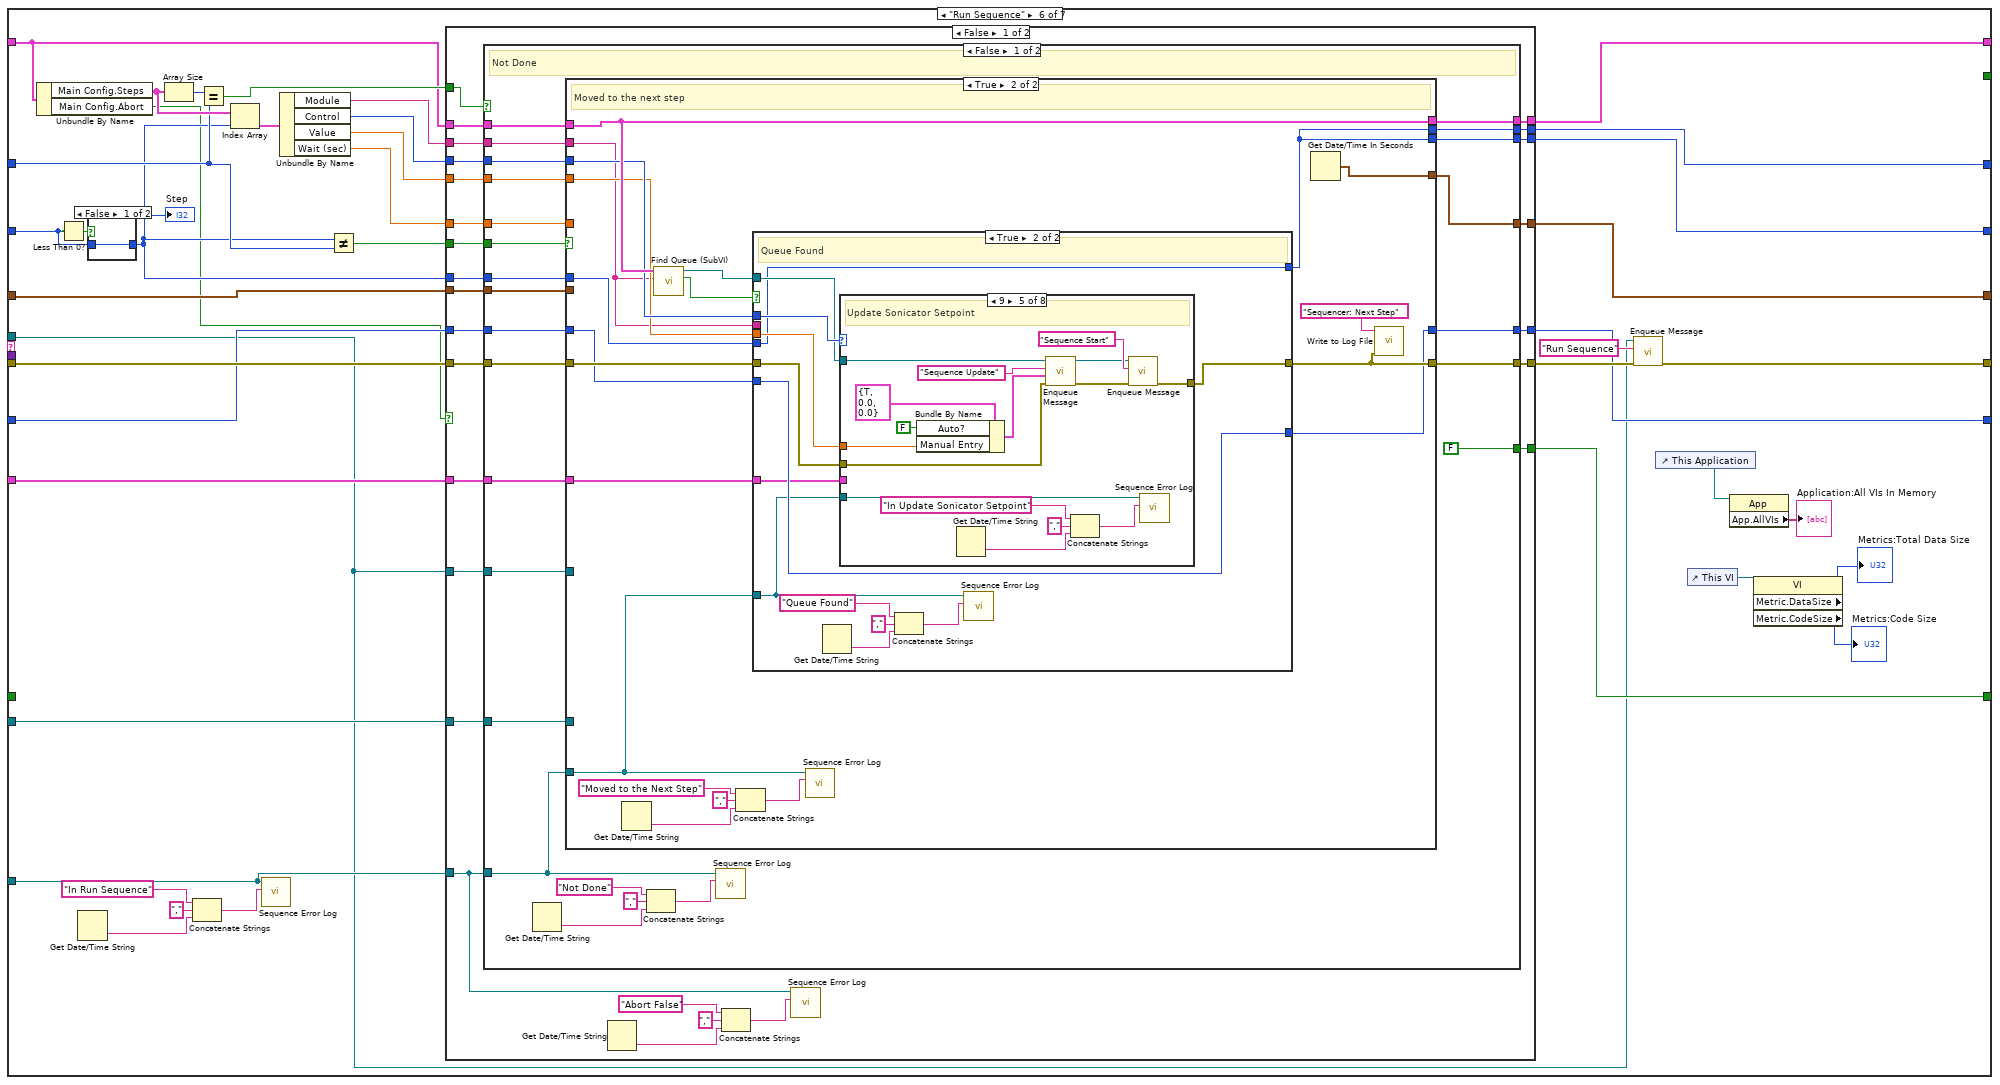
[diagram p13: hidden frame]
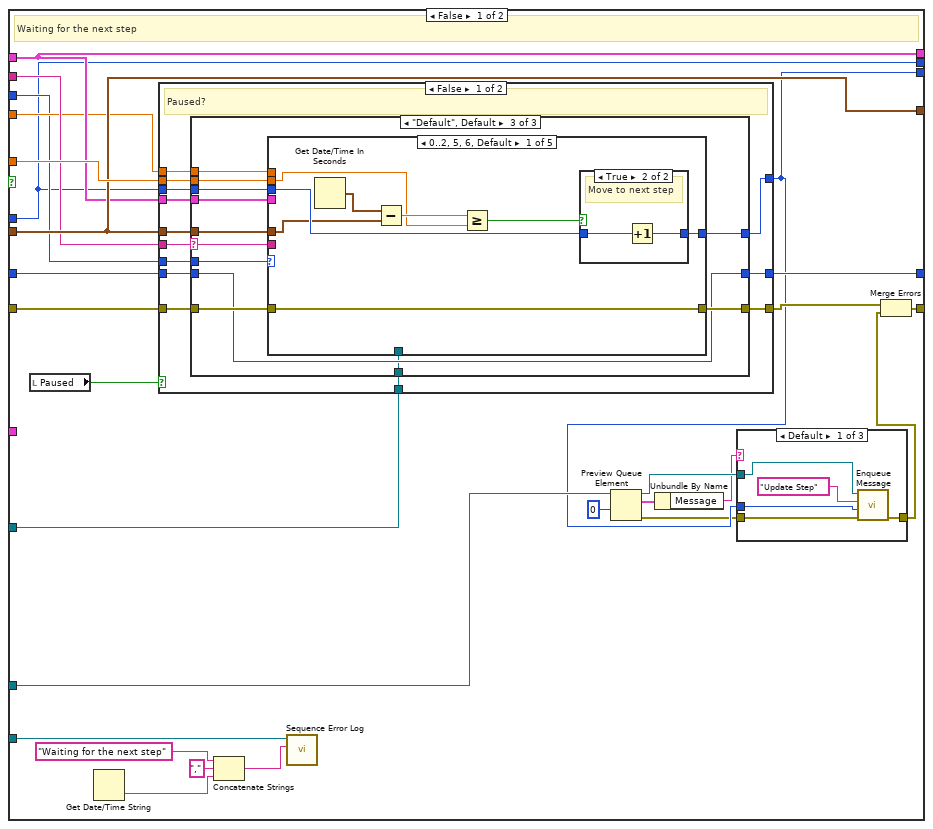
[diagram p14: hidden frame]
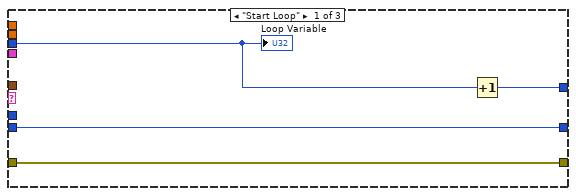
[diagram p17: hidden frame]
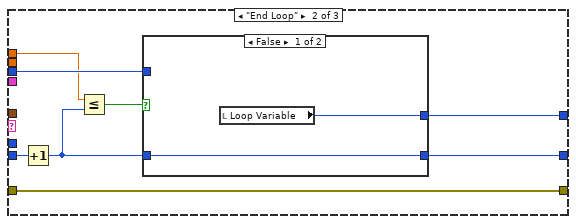
[diagram p18: hidden frame]
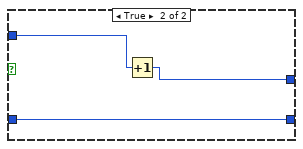
[diagram p19: hidden frame]
diagram:
  # "Loop Count"
  # "This step"
  # "Last Step"
  n1 = flat-sequence {
    tunnel: [w20] -> w15
    tunnel: [w32] -> w7
    tunnel: "error in (no error)" -> [w20]
    frame #0 {
      w38 = FALSE ("Paused")
      n2 = local write "Stop"(w38) -> ()
      n3 = local write "Done"(w38) -> ()
      n4 = local write "Paused"(w38) -> ()
      n5 = Get Date/Time String() -> (date string=w31:string, time string=w26:string)  [unwired: 3 in]
      n6 = Search and Replace String(replace all?=TRUE ("replace all? (F)"), input string=w31, search string="/", replace string="_" ("replace string (\"\")")) -> (result string=w22:string)  [unwired: 4 in, 3 out]
      n7 = Search and Replace String(replace all?=TRUE ("replace all? (F)"), input string=w26, search string=":", replace string="_" ("replace string (\"\")")) -> (result string=w21:string)  [unwired: 4 in, 3 out]
      n8 = Concatenate Strings("Sequence Log " ("string"), w22, w21) -> (w37:string)
      n9 = Build Path(base path=path "C:/Users/Public/Documents/Sequence Crash Error Log", name or relative path=w37) -> (appended path=w36:path)
      n10 = Open/Create/Replace File(file path (use dialog)=w36, operation (0:open)=T75."open or create") -> (refnum out=w32:refnum<file>, error out=→"error out 2":errorcluster)  [unwired: 4 in, 1 out]
    }
  }
  n11 = Unbundle By Name("Message Queues in") -> ("Sequence"=w18:refnum<queue>, "Sequence UI"=w9:refnum<queue>)
  n12 = call "Obtain Message Queue.vi"("name (unnamed)"="Sequence Loop") -> ("Message Queue"=w16:refnum<queue>)  [unwired: 9 in, 1 out]
  n13 = while {
    tunnel: w18 -> [w41]
    tunnel: w15 -> [w44]
    tunnel: [w45] -> w14
    tunnel: w16 -> [w40]
    tunnel: [w39] -> w4
    stop <- w42 stop-if-true
    n14 = call "Dequeue Message.vi"("error in (no error)"=w44, "Message Queue"=w41) -> ("error out"=w43:errorcluster, "Message Data"=w46:variant, "Message"=w47:string, "dup Message Queue"=w39:refnum<queue>)  [unwired: 6 in]
    n15 = case shown="\"Update Sequence\"" w47 {
      tunnel: w46 -> [_ _ _ _ w66 w71 w76]
      tunnel: w43 -> [w48 w55 w59 w64 w68 w73 w78]
      tunnel: [w48 w49 w58 w63 w67 w72 w77] -> w45
      tunnel: [_ _ w56 w61 _ _ _] -> w42
      tunnel: w40 -> [_ w53 w57 w62 w69 w74 w79]
      frame Default {
      }
      frame "Start Sequence" {
        n16 = call-poly "Enqueue Message.vi"("error in (no error)"=w55, "Message"="Send Settings", "Message Queue"=w53) -> ("error out"=w50:errorcluster, "dup Message Queue"=w52:refnum<queue>)  [unwired: 7 in]
        n17 = call-poly "Enqueue Message.vi"("error in (no error)"=w50, "Message"="Run Sequence", "Message Queue"=w52) -> ("error out"=w49:errorcluster)  [unwired: 7 in, 1 out]
      }
      frame "E-Stop", "Stop" {
        w56 = FALSE
        n18 = call-poly "Enqueue Message.vi"("error in (no error)"=w59, "Message"="Pause", "Message Queue"=w57) -> ("error out"=w58:errorcluster)  [unwired: 7 in, 1 out]
        "Stop" <- w56
      }
      frame "Exit" {
        w61 = TRUE
        n19 = call-poly "Enqueue Message.vi"("error in (no error)"=w64, "Message"="Exit", "Message Queue"=w62) -> ("error out"=w63:errorcluster)  [unwired: 7 in, 1 out]
        n20 = local write "Stop"(w61) -> ()
      }
      frame "Update Sequence" {
        n21 = call-poly "Enqueue Message.vi"("error in (no error)"=w68, "Message Data"=w66, "Message"="Update Sequence", "Message Queue"=w69) -> ("error out"=w67:errorcluster)  [unwired: 6 in, 1 out]
      }
      frame "Pause Sequence" {
        n22 = call-poly "Enqueue Message.vi"("error in (no error)"=w73, "Message Data"=w71, "Message"="Pause", "Message Queue"=w74) -> ("error out"=w72:errorcluster)  [unwired: 6 in, 1 out]
      }
      frame "Resume Sequence" {
        n23 = call-poly "Enqueue Message.vi"("error in (no error)"=w78, "Message Data"=w76, "Message"="Resume", "Message Queue"=w79) -> ("error out"=w77:errorcluster)  [unwired: 6 in, 1 out]
      }
    }
  }
  n24 = while {
    tunnel: w16 -> [w82]
    tunnel: w15 -> [w105]
    shift-right: [w102] -> _
    shift-left: "Input 2" -> [w92]
    tunnel: [w100] -> w12
    shift-right: [w95] -> _
    shift-left: -1 -> [w97]
    shift-right: [w94] -> _
    shift-left: _ -> [w96]
    shift-right: [w90] -> _
    shift-left: -1 -> [w91]
    shift-right: [w89] -> _
    shift-left: _ -> [w88]
    tunnel: w9 -> [w81]
    shift-right: [w87] -> _
    shift-left: 0 -> [w86]
    tunnel: w7 -> [w84]
    tunnel: T74 {"Auto?"=TRUE, "Manual Entry"=0.0, "Setpoint"=0.0} -> [w83]
    tunnel: [w82] -> w3
    tunnel: [w81] -> w2
    stop <- w99 stop-if-true
    n25 = call "Dequeue Message.vi"("error in (no error)"=w105, "timeout in ms (-1)"=1, "Message Queue"=w82) -> ("error out"=w101:errorcluster, "Message Data"=w103:variant, "Message"=w104:string, "dup Message Queue"=w93:refnum<queue>)  [unwired: 5 in]
    n26 = Wait (ms)(milliseconds to wait=u32 5) -> ()  [unwired: 1 out]
    n27 = case shown="\"Update Sequence\"" w104 {
      tunnel: w103 -> [_ w133 _ _ _ _ _]
      tunnel: [w115 w123 w142 w206 w217 w257 w720] -> w102
      tunnel: w101 -> [w114 w132 w136 w199 w210 w256 w719]
      tunnel: [w114 w125 w138 w199 w210 w245 w719] -> w100
      tunnel: [_ _ _ _ _ _ TRUE] -> w99
      tunnel: w92 -> [w115 _ w142 w206 w217 w239 w720]
      tunnel: w97 -> [w113 w130 _ w204 w215 w242 w718]
      tunnel: w96 -> [w112 w129 w143 w205 w216 w236 w717]
      tunnel: w91 -> [w110 w128 _ w202 w213 w248 w716]
      tunnel: [w113 w130 w140 w204 w215 w254 w718] -> w95
      tunnel: [w112 w129 w143 w205 w216 w251 w717] -> w94
      tunnel: w93 -> [_ _ _ _ _ w218 _]
      tunnel: [w110 w128 w140 w202 w213 w241 w716] -> w90
      tunnel: [w109 w127 FALSE w201 w212 w235 w715] -> w89
      tunnel: w88 -> [w109 w127 _ w201 w212 _ w715]
      tunnel: w81 -> [_ _ _ _ _ w233 _]
      tunnel: [w108 w124 w137 w198 w209 w232 w714] -> w87
      tunnel: w86 -> [w108 w124 w137 w198 w209 w231 w714]
      tunnel: w84 -> [w107 w116 w134 w196 w207 w225 w712]
      tunnel: w83 -> [_ _ _ _ _ w224 _]
      frame Default {
        n28 = call "Sequence Error Log.vi"("string"="In Default", "Byte Stream File in"=w107) -> ()  [unwired: 10 in]
        n29 = Wait (ms)(milliseconds to wait=u32 1000) -> ()  [unwired: 1 out]
      }
      frame "Update Sequence" {
        n30 = call "Sequence Error Log.vi"("string"="In Update Sequence", "Byte Stream File in"=w116) -> ()  [unwired: 10 in]
        n31 = Variant To Data(error in=w132, type="Input", Variant=w133) -> (data=w123:T1, error out=w125:errorcluster)
        "Output" <- w123
        n32 = Unbundle By Name(w123) -> ("Main Config.Pump Module Configs"=w122:T44[])
        n33 = Index Array(array=w122, index=0) -> (element=w120:T44)
        n34 = Unbundle By Name(w120) -> ("Process Name"=→"Process Name":string, "Queue Name"=→"Queue Name":string)
        n35 = call "Write to Log File.vi"("error in"=w125, "text"="Sequencer: Update") -> ()  [unwired: 9 in, 1 out]
      }
      frame "Send Settings" {
        w140 = -1
        n36 = Unbundle By Name(w142) -> ("Main Config.Steps"=w145:T57)
        n37 = call "Sequence Error Log.vi"("string"="In Send Settings", "Byte Stream File in"=w134) -> ()  [unwired: 10 in]
        n38 = for {
          tunnel: w145 -> [w154] mode=indexing
          tunnel: [w149] -> w144 mode=indexing
          tunnel: w136 -> [w151]
          tunnel: w142 -> [w148]
          n39 = Unbundle By Name(w154) -> ("Module"=w153:string, "Control"=w146:u16, "Value"=w155:dbl)
          n40 = call "Find Queue (SubVI).vi"("Module"=w153, "Input"=w148) -> ("Found?"=w152:bool, "Queue out"=w147:refnum<queue>)  [unwired: 8 in]
          n41 = case shown="1, 5, 6, 9" w146 {
            tunnel: [w189 w193] -> w150
            tunnel: w155 -> [w188 w192]
            frame 0, Default {
              n42 = Bundle By Name(cluster=T74 {"Auto?"=TRUE, "Manual Entry"=0.0, "Setpoint"=0.0}, "Auto?"=FALSE, "Manual Entry"=w188) -> (w189:T74)
            }
            frame 1, 5, 6, 9 {
              n43 = Bundle By Name(cluster=T74 {"Auto?"=TRUE, "Manual Entry"=0.0, "Setpoint"=0.0}, "Auto?"=TRUE, "Setpoint"=w192) -> (w193:T74)
            }
          }
          n44 = case shown="True" w152 {
            tunnel: w151 -> [w156 w161]
            tunnel: w150 -> [_ w160]
            tunnel: [w156 w159] -> w149
            tunnel: w147 -> [_ w158]
            tunnel: w146 -> [_ w157]
            frame False {
            }
            frame True {
              n45 = case shown="Default" w157 {
                tunnel: w161 -> [w166 w167 w171 w181]
                tunnel: w160 -> [w165 _ w170 w180]
                tunnel: [w163 w167 w169 w179] -> w159
                tunnel: w158 -> [w162 _ w168 w178]
                frame Default {
                  n46 = call-poly "Enqueue Message.vi"("error in (no error)"=w166, "Message Data"=w165, "Message"="Sequence Update", "Message Queue"=w162) -> ("error out"=w163:errorcluster)  [unwired: 6 in, 1 out]
                }
                frame 3, 4, 7, 8 {
                }
                frame 5 {
                  n47 = disable-structure shown="Disabled" {
                    disable-tunnel: w171 -> [w176 w177]
                    disable-tunnel: w170 -> [w175 _]
                    disable-tunnel: [w173 w177] -> w169
                    disable-tunnel: w168 -> [w172 _]
                    frame Disabled {
                      n48 = call-poly "Enqueue Message.vi"("error in (no error)"=w176, "Message Data"=w175, "Message"="Sequence Update Speed", "Message Queue"=w172) -> ("error out"=w173:errorcluster)  [unwired: 6 in, 1 out]
                    }
                    frame Enabled {
                    }
                  }
                }
                frame 6 {
                  n49 = disable-structure shown="Enabled" {
                    disable-tunnel: w181 -> [w186 w187]
                    disable-tunnel: w180 -> [w185 _]
                    disable-tunnel: [w183 w187] -> w179
                    disable-tunnel: w178 -> [w182 _]
                    frame Disabled {
                      n50 = call-poly "Enqueue Message.vi"("error in (no error)"=w186, "Message Data"=w185, "Message"="Sequence Update Temperature", "Message Queue"=w182) -> ("error out"=w183:errorcluster)  [unwired: 6 in, 1 out]
                    }
                    frame Enabled {
                    }
                  }
                }
              }
            }
          }
          "Intruction Cluster" <- w154
        }
        n51 = Merge Errors(w136, w144) -> (w138:errorcluster)
        n52 = call "Write to Log File.vi"("error in"=w138, "text"="Sequencer: Send Settings") -> ()  [unwired: 9 in, 1 out]
      }
      frame "Pause" {
        n53 = call "Sequence Error Log.vi"("string"="In Pause", "Byte Stream File in"=w196) -> ()  [unwired: 10 in]
        n54 = call "Write to Log File.vi"("error in"=w199, "text"="Sequencer: Pause") -> ()  [unwired: 9 in, 1 out]
        "Paused" <- TRUE ("Paused")
      }
      frame "Resume" {
        n55 = call "Sequence Error Log.vi"("string"="In Resume", "Byte Stream File in"=w207) -> ()  [unwired: 10 in]
        n56 = local write "Paused"(FALSE ("Paused")) -> ()
        n57 = call "Write to Log File.vi"("error in"=w210, "text"="Sequencer: Resume") -> ()  [unwired: 9 in, 1 out]
      }
      frame "Run Sequence" {
        n58 = Unbundle By Name(w239) -> ("Main Config.Steps"=w250:T57, "Main Config.Abort"=w230:bool)
        n59 = Less Than 0?(x=w242) -> (x < 0?=w243:bool)
        n60 = Get Date/Time String() -> (time string=w227:string)  [unwired: 3 in, 1 out]
        n61 = case shown="False" w243 {
          tunnel: [w710 0] -> w234
          tunnel: w242 -> [w710 _]
          frame False {
          }
          frame True {
          }
        }
        "Step" <- w234
        n62 = Array Size(array=w250) -> (size(s)=w249:i32)
        n63 = Concatenate Strings("In Run Sequence" ("string"), "," ("string"), w227) -> (w226:string)
        n64 = Equal?(x=w249, y=w248) -> (x = y?=w247:bool)
        n65 = Index Array(array=w250, index=w234) -> (element=w253:T58)
        n66 = call "Sequence Error Log.vi"("string"=w226, "Byte Stream File in"=w225) -> ()  [unwired: 10 in]
        n67 = Unbundle By Name(w253) -> ("Module"=w252:string, "Control"=w238:u16, "Value"=w237:dbl, "Wait (sec)"=w240:dbl)
        n68 = Not Equal?(x=w234, y=w248) -> (x != y?=w255:bool)
        n69 = case shown="False" w230 {
          tunnel: [w283 w701] -> w257
          tunnel: w256 -> [w282 w703]
          tunnel: w255 -> [w281 _]
          tunnel: [w280 w699] -> w254
          tunnel: w252 -> [w279 _]
          tunnel: [w278 w704] -> w251
          tunnel: w247 -> [w277 _]
          tunnel: [w276 w703] -> w246
          tunnel: [w275 w699] -> w241
          tunnel: w240 -> [w274 _]
          tunnel: w239 -> [w273 w701]
          tunnel: w238 -> [w272 _]
          tunnel: w237 -> [w271 _]
          tunnel: w236 -> [w270 w704]
          tunnel: [w269 TRUE] -> w235
          tunnel: w234 -> [w268 _]
          tunnel: w233 -> [w267 _]
          tunnel: [w266 0] -> w232
          tunnel: w231 -> [w265 _]
          tunnel: w225 -> [w260 w691]
          tunnel: w224 -> [w259 _]
          tunnel: w218 -> [w258 _]
          frame False {
            n70 = case shown="False" w277 {
              tunnel: [w308 w685] -> w283
              tunnel: w282 -> [w299 w679]
              tunnel: w273 -> [w307 w685]
              tunnel: [w306 w679] -> w276
              tunnel: w281 -> [w305 _]
              tunnel: w268 -> [w304 w683]
              tunnel: [w303 w683] -> w280
              tunnel: w279 -> [w302 _]
              tunnel: w274 -> [w301 _]
              tunnel: [w300 w682] -> w278
              tunnel: [w298 w683] -> w275
              tunnel: w272 -> [w297 _]
              tunnel: w271 -> [w296 _]
              tunnel: w270 -> [w295 w682]
              tunnel: [FALSE w681] -> w269
              tunnel: w267 -> [w293 _]
              tunnel: [w292 0] -> w266
              tunnel: w265 -> [w291 _]
              tunnel: w260 -> [w286 w673]
              tunnel: w259 -> [w285 _]
              tunnel: w258 -> [w284 _]
              frame False {
                # "Not Done"
                n71 = Get Date/Time String() -> (time string=w288:string)  [unwired: 3 in, 1 out]
                n72 = case shown="True" w305 {
                  tunnel: [w332 w515] -> w308
                  tunnel: w304 -> [w327 w505]
                  tunnel: w307 -> [w332 w515]
                  tunnel: [w325 w507] -> w306
                  tunnel: [w314 w504] -> w303
                  tunnel: w302 -> [w331 w506]
                  tunnel: w301 -> [w335 _]
                  tunnel: [w333 w509] -> w300
                  tunnel: w299 -> [w330 w512]
                  tunnel: [w327 w504] -> w298
                  tunnel: w297 -> [w328 w511]
                  tunnel: w296 -> [w329 w510]
                  tunnel: w295 -> [w333 _]
                  tunnel: w293 -> [w316 _]
                  tunnel: [w324 w502] -> w292
                  tunnel: w291 -> [w323 w503]
                  tunnel: w286 -> [w318 w497]
                  tunnel: w285 -> [_ w496]
                  tunnel: w284 -> [w317 _]
                  frame False {
                    # "Waiting for the next step"
                    n73 = local read "Paused"() -> (w334:bool)
                    n74 = Get Date/Time String() -> (time string=w320:string)  [unwired: 3 in, 1 out]
                    n75 = case shown="False" w334 {
                      tunnel: [w355 w495] -> w314
                      tunnel: w327 -> [w354 w495]
                      tunnel: w335 -> [w353 _]
                      tunnel: w333 -> [w352 _]
                      tunnel: w328 -> [w351 _]
                      tunnel: w332 -> [w350 _]
                      tunnel: w331 -> [w346 _]
                      tunnel: w330 -> [w349 w494]
                      tunnel: [w348 w494] -> w326
                      tunnel: w329 -> [w347 _]
                      tunnel: [w345 w493] -> w324
                      tunnel: w323 -> [w344 w493]
                      tunnel: w317 -> [w343 _]
                      frame False {
                        # "Paused?"
                        n76 = case shown="\"Default\", Default" w346 {
                          selector: w346 -> [_ _ w375]
                          tunnel: [w357 w367 w384] -> w355
                          tunnel: w354 -> [w358 w365 w383]
                          tunnel: w353 -> [_ _ w382]
                          tunnel: w352 -> [_ _ w381]
                          tunnel: w351 -> [_ _ w380]
                          tunnel: w350 -> [_ _ w379]
                          tunnel: w349 -> [w359 w366 w378]
                          tunnel: [w359 w366 w377] -> w348
                          tunnel: w347 -> [_ w363 w376]
                          tunnel: [w356 w362 w374] -> w345
                          tunnel: w344 -> [w356 w361 w374]
                          tunnel: w343 -> [_ _ w373]
                          frame "Start Loop" {
                            n77 = Increment(x=w358) -> (x+1=w357:u32)
                            "Loop Variable" <- w358
                          }
                          frame "End Loop" {
                            n78 = Increment(x=w361) -> (x+1=w360:i32)
                            n79 = Less Or Equal?(x=w363, y=w360) -> (x <= y?=w364:bool)
                            n80 = case shown="False" w364 {
                              tunnel: [w369 w371] -> w367
                              tunnel: w365 -> [_ w372]
                              tunnel: [w368 w370] -> w362
                              tunnel: w360 -> [w368 w370]
                              frame False {
                                n81 = local read "Loop Variable"() -> (w369:u32)
                              }
                              frame True {
                                n82 = Increment(x=w372) -> (x+1=w371:u32)
                              }
                            }
                          }
                          frame "Default", Default {
                            n83 = case shown="0..2, 5, 6, Default" w380 {
                              tunnel: [w389 w405 w429 w453 w477] -> w384
                              tunnel: w383 -> [w388 w404 w428 w452 w476]
                              tunnel: w382 -> [w387 _ _ _ _]
                              tunnel: w381 -> [w386 _ _ _ _]
                              tunnel: w379 -> [_ w403 w427 w451 w475]
                              tunnel: w375 -> [_ w402 w426 w450 w474]
                              tunnel: w378 -> [w385 w399 w423 w447 w471]
                              tunnel: [w385 w398 w422 w446 w470] -> w377
                              tunnel: w376 -> [_ w397 w421 w445 w469]
                              tunnel: w373 -> [_ w396 w420 w444 w468]
                              frame 0..2, 5, 6, Default {
                                n84 = Get Date/Time In Seconds() -> (seconds since 1Jan1904=w392:timestamp)
                                n85 = Subtract(x=w392, y=w386) -> (x-y=w390:dbl)
                                n86 = Greater Or Equal?(x=w390, y=w387) -> (x >= y?=w391:bool)
                                n87 = case shown="True" w391 {
                                tunnel: w388 -> [w393 w395]
                                tunnel: [w393 w394] -> w389
                                frame False {
                                }
                                frame True {
                                # "Move to next step"
                                n88 = Increment(x=w395) -> (x+1=w394:u32)
                                }
                                }
                              }
                              frame 3 {
                                # "Wait Until Less Than"
                                n89 = call "Find Queue (SubVI).vi"("Module"=w402, "Input"=w403) -> ("Found?"=w401:bool, "Queue out"=w400:refnum<queue>)  [unwired: 8 in]
                                n90 = case shown="True" w401 {
                                tunnel: [w407 w416] -> w405
                                tunnel: w404 -> [w407 w415]
                                tunnel: w400 -> [_ w414]
                                tunnel: w399 -> [w406 w413]
                                tunnel: [w406 w412] -> w398
                                tunnel: w397 -> [_ w410]
                                tunnel: w396 -> [_ w408]
                                frame False {
                                # "Error"
                                }
                                frame True {
                                n91 = call "Get Wait Until Data.vi"("error in (no error)"=w413, "Sequence Data Queue"=w408, "Queue in"=w414) -> ("error out"=w412:errorcluster, "Data"=w411:dbl)  [unwired: 7 in]
                                n92 = Less Or Equal?(x=w411, y=w410) -> (x <= y?=w409:bool)
                                n93 = case shown="True" w409 {
                                tunnel: w415 -> [w417 w419]
                                tunnel: [w417 w418] -> w416
                                frame False {
                                }
                                frame True {
                                # "Move to next step"
                                n94 = Increment(x=w419) -> (x+1=w418:u32)
                                }
                                }
                                }
                                }
                              }
                              frame 4 {
                                # "Wait Until Greater Than"
                                n95 = call "Find Queue (SubVI).vi"("Module"=w426, "Input"=w427) -> ("Found?"=w425:bool, "Queue out"=w424:refnum<queue>)  [unwired: 8 in]
                                n96 = case shown="True" w425 {
                                tunnel: [w431 w440] -> w429
                                tunnel: w428 -> [w431 w439]
                                tunnel: w424 -> [_ w438]
                                tunnel: w423 -> [w430 w437]
                                tunnel: [w430 w436] -> w422
                                tunnel: w421 -> [_ w434]
                                tunnel: w420 -> [_ w432]
                                frame False {
                                # "Error"
                                }
                                frame True {
                                n97 = call "Get Wait Until Data.vi"("error in (no error)"=w437, "Sequence Data Queue"=w432, "Queue in"=w438) -> ("error out"=w436:errorcluster, "Data"=w435:dbl)  [unwired: 7 in]
                                n98 = Greater Or Equal?(x=w435, y=w434) -> (x >= y?=w433:bool)
                                n99 = case shown="True" w433 {
                                tunnel: w439 -> [w441 w443]
                                tunnel: [w441 w442] -> w440
                                frame False {
                                }
                                frame True {
                                # "Move to next step"
                                n100 = Increment(x=w443) -> (x+1=w442:u32)
                                }
                                }
                                }
                                }
                              }
                              frame 7 {
                                # "Wait Until TCU is Less Than"
                                n101 = call "Find Queue (SubVI).vi"("Module"=w450, "Input"=w451) -> ("Found?"=w449:bool, "Queue out"=w448:refnum<queue>)  [unwired: 8 in]
                                n102 = case shown="True" w449 {
                                tunnel: [w455 w464] -> w453
                                tunnel: w452 -> [w455 w463]
                                tunnel: w448 -> [_ w462]
                                tunnel: w447 -> [w454 w461]
                                tunnel: [w454 w460] -> w446
                                tunnel: w445 -> [_ w458]
                                tunnel: w444 -> [_ w456]
                                frame False {
                                # "Error"
                                }
                                frame True {
                                n103 = call "Get Wait Until Data.vi"("error in (no error)"=w461, "Sequence Data Queue"=w456, "Queue in"=w462) -> ("error out"=w460:errorcluster, "Data"=w459:dbl)  [unwired: 7 in]
                                n104 = Less Or Equal?(x=w459, y=w458) -> (x <= y?=w457:bool)
                                n105 = case shown="True" w457 {
                                tunnel: w463 -> [w465 w467]
                                tunnel: [w465 w466] -> w464
                                frame False {
                                }
                                frame True {
                                # "Move to next step"
                                n106 = Increment(x=w467) -> (x+1=w466:u32)
                                }
                                }
                                }
                                }
                              }
                              frame 8 {
                                # "Wait Until TCU is Greater Than"
                                n107 = call "Find Queue (SubVI).vi"("Module"=w474, "Input"=w475) -> ("Found?"=w473:bool, "Queue out"=w472:refnum<queue>)  [unwired: 8 in]
                                n108 = case shown="True" w473 {
                                tunnel: [w479 w488] -> w477
                                tunnel: w476 -> [w479 w487]
                                tunnel: w472 -> [_ w486]
                                tunnel: w471 -> [w478 w485]
                                tunnel: [w478 w484] -> w470
                                tunnel: w469 -> [_ w482]
                                tunnel: w468 -> [_ w480]
                                frame False {
                                # "Error"
                                }
                                frame True {
                                n109 = call "Get Wait Until Data.vi"("error in (no error)"=w485, "Sequence Data Queue"=w480, "Queue in"=w486) -> ("error out"=w484:errorcluster, "Data"=w483:dbl)  [unwired: 7 in]
                                n110 = Greater Or Equal?(x=w483, y=w482) -> (x >= y?=w481:bool)
                                n111 = case shown="True" w481 {
                                tunnel: w487 -> [w489 w491]
                                tunnel: [w489 w490] -> w488
                                frame False {
                                }
                                frame True {
                                # "Move to next step"
                                n112 = Increment(x=w491) -> (x+1=w490:u32)
                                }
                                }
                                }
                                }
                              }
                            }
                          }
                        }
                      }
                      frame True {
                        # "Paused?"
                        n113 = Wait (ms)(milliseconds to wait=u32 50) -> ()  [unwired: 1 out]
                      }
                    }
                    n114 = Concatenate Strings("Waiting for the next step" ("string"), "," ("string"), w320) -> (w319:string)
                    n115 = call "Sequence Error Log.vi"("string"=w319, "Byte Stream File in"=w318) -> ()  [unwired: 10 in]
                    n116 = Preview Queue Element(queue=w316, timeout in ms (-1)=0) -> (queue out=w313:refnum<queue>, element=w311:T76, error out=w309:errorcluster)  [unwired: 1 in, 1 out]
                    n117 = Unbundle By Name(w311) -> ("Message"=w310:string)
                    n118 = case shown="Default" w310 {
                      tunnel: w314 -> [w336 _ _]
                      tunnel: w313 -> [w337 _ _]
                      tunnel: [w338 w341 w342] -> w312
                      tunnel: w309 -> [w339 w341 w342]
                      frame Default {
                        n119 = call-poly "Enqueue Message.vi"("error in (no error)"=w339, "Message Data"=w336, "Message"="Update Step", "Message Queue"=w337) -> ("error out"=w338:errorcluster)  [unwired: 6 in, 1 out]
                      }
                      frame "Update Step" {
                      }
                      frame "Exit" {
                      }
                    }
                    n120 = Merge Errors(w326, w312) -> (w325:errorcluster)
                  }
                  frame True {
                    # "Moved to the next step"
                    n121 = Get Date/Time String() -> (time string=w499:string)  [unwired: 3 in, 1 out]
                    n122 = call "Find Queue (SubVI).vi"("Module"=w506, "Input"=w515) -> ("Found?"=w514:bool, "Queue out"=w513:refnum<queue>)  [unwired: 8 in]
                    n123 = Concatenate Strings("Moved to the Next Step" ("string"), "," ("string"), w499) -> (w498:string)
                    n124 = case shown="True" w514 {
                      tunnel: w513 -> [_ w558]
                      tunnel: w512 -> [w527 w557]
                      tunnel: [w526 w556] -> w507
                      tunnel: w511 -> [_ w560]
                      tunnel: w510 -> [w522 w559]
                      tunnel: w506 -> [w528 _]
                      tunnel: w505 -> [w525 w555]
                      tunnel: [w524 w555] -> w504
                      tunnel: w503 -> [w523 w554]
                      tunnel: [w521 w554] -> w502
                      tunnel: w497 -> [w516 w549]
                      tunnel: w496 -> [_ w548]
                      frame False {
                        # "Queue not found. ERROR"
                        n125 = Get Date/Time String() -> (time string=w518:string)  [unwired: 3 in, 1 out]
                        n126 = case shown="\"End Loop\"" w528 {
                          tunnel: [w531 w538 w547] -> w526
                          tunnel: w527 -> [w531 w538 w547]
                          tunnel: w525 -> [w530 w534 w546]
                          tunnel: [w530 w539 w546] -> w524
                          tunnel: w523 -> [w529 w536 w545]
                          tunnel: w522 -> [_ w537 _]
                          tunnel: [w529 w533 w545] -> w521
                          frame "Start Loop" {
                            n127 = local write "Loop Variable"(w530) -> ()
                          }
                          frame "End Loop" {
                            n128 = Increment(x=w536) -> (x+1=w532:i32)
                            n129 = Less Or Equal?(x=w537, y=w532) -> (x <= y?=w535:bool)
                            n130 = case shown="True" w535 {
                              tunnel: [w541 w543] -> w539
                              tunnel: w534 -> [_ w544]
                              tunnel: [w540 0] -> w533
                              tunnel: w532 -> [w540 _]
                              frame False {
                                n131 = local read "Loop Variable"() -> (w541:u32)
                              }
                              frame True {
                                n132 = Increment(x=w544) -> (x+1=w543:u32)
                              }
                            }
                          }
                          frame "Default", Default {
                            # "Error"
                          }
                        }
                        n133 = Concatenate Strings("Queue Not Found" ("string"), "," ("string"), w518) -> (w517:string)
                        n134 = call "Sequence Error Log.vi"("string"=w517, "Byte Stream File in"=w516) -> ()  [unwired: 10 in]
                      }
                      frame True {
                        # "Queue Found"
                        n135 = Get Date/Time String() -> (time string=w551:string)  [unwired: 3 in, 1 out]
                        n136 = case shown="9" w560 {
                          tunnel: w559 -> [w574 w591 w606 w622 w638 w653 _ _]
                          tunnel: w558 -> [w572 w588 w603 w619 w635 w651 _ w669]
                          tunnel: w557 -> [w570 w587 w602 w618 w634 w652 w661 w668]
                          tunnel: [w566 w583 w598 w614 w630 w646 w661 w667] -> w556
                          tunnel: w549 -> [w561 w578 w593 w609 w625 w641 w656 w662]
                          tunnel: w548 -> [_ w577 _ _ _ _ _ _]
                          frame 0 {
                            # "Manual"
                            n137 = Get Date/Time String() -> (time string=w563:string)  [unwired: 3 in, 1 out]
                            n138 = Bundle By Name(cluster=T74 {"Auto?"=TRUE, "Manual Entry"=0.0, "Setpoint"=0.0}, "Auto?"=FALSE, "Manual Entry"=w574) -> (w571:T74)
                            n139 = Concatenate Strings("In Manual" ("string"), "," ("string"), w563) -> (w562:string)
                            n140 = call-poly "Enqueue Message.vi"("error in (no error)"=w570, "Message Data"=w571, "Message"="Sequence Update", "Message Queue"=w572) -> ("error out"=w568:errorcluster, "dup Message Queue"=w569:refnum<queue>)  [unwired: 6 in]
                            n141 = call "Sequence Error Log.vi"("string"=w562, "Byte Stream File in"=w561) -> ()  [unwired: 10 in]
                            n142 = call-poly "Enqueue Message.vi"("error in (no error)"=w568, "Message"="Sequence Start", "Message Queue"=w569) -> ("error out"=w566:errorcluster)  [unwired: 7 in, 1 out]
                          }
                          frame 1 {
                            # "Auto"
                            n143 = Get Date/Time String() -> (time string=w580:string)  [unwired: 3 in, 1 out]
                            n144 = Bundle By Name(cluster=w577, "Auto?"=TRUE, "Setpoint"=w591) -> (w589:T74)
                            n145 = Concatenate Strings("In Auto" ("string"), "," ("string"), w580) -> (w579:string)
                            n146 = call-poly "Enqueue Message.vi"("error in (no error)"=w587, "Message Data"=w589, "Message"="Sequence Update", "Message Queue"=w588) -> ("error out"=w585:errorcluster, "dup Message Queue"=w584:refnum<queue>)  [unwired: 6 in]
                            n147 = call "Sequence Error Log.vi"("string"=w579, "Byte Stream File in"=w578) -> ()  [unwired: 10 in]
                            n148 = call-poly "Enqueue Message.vi"("error in (no error)"=w585, "Message"="Sequence Start", "Message Queue"=w584) -> ("error out"=w583:errorcluster)  [unwired: 7 in, 1 out]
                          }
                          frame 5 {
                            # "Update TCU Speed"
                            n149 = Get Date/Time String() -> (time string=w595:string)  [unwired: 3 in, 1 out]
                            n150 = Bundle By Name(cluster=T74 {"Auto?"=TRUE, "Manual Entry"=0.0, "Setpoint"=0.0}, "Auto?"=TRUE, "Setpoint"=w606) -> (w604:T74)
                            n151 = Concatenate Strings("Update TCU Speed" ("string"), "," ("string"), w595) -> (w594:string)
                            n152 = call-poly "Enqueue Message.vi"("error in (no error)"=w602, "Message Data"=w604, "Message"="Sequence Update Speed", "Message Queue"=w603) -> ("error out"=w600:errorcluster, "dup Message Queue"=w599:refnum<queue>)  [unwired: 6 in]
                            n153 = call "Sequence Error Log.vi"("string"=w594, "Byte Stream File in"=w593) -> ()  [unwired: 10 in]
                            n154 = call-poly "Enqueue Message.vi"("error in (no error)"=w600, "Message"="Sequence Start", "Message Queue"=w599) -> ("error out"=w598:errorcluster)  [unwired: 7 in, 1 out]
                          }
                          frame 6 {
                            # "Update TCU Tempurature"
                            n155 = Get Date/Time String() -> (time string=w611:string)  [unwired: 3 in, 1 out]
                            n156 = Bundle By Name(cluster=T74 {"Auto?"=TRUE, "Manual Entry"=0.0, "Setpoint"=0.0}, "Auto?"=TRUE, "Setpoint"=w622) -> (w620:T74)
                            n157 = Concatenate Strings("In Update TCU Temp" ("string"), "," ("string"), w611) -> (w610:string)
                            n158 = call-poly "Enqueue Message.vi"("error in (no error)"=w618, "Message Data"=w620, "Message"="Sequence Update Temperature", "Message Queue"=w619) -> ("error out"=w616:errorcluster, "dup Message Queue"=w615:refnum<queue>)  [unwired: 6 in]
                            n159 = call "Sequence Error Log.vi"("string"=w610, "Byte Stream File in"=w609) -> ()  [unwired: 10 in]
                            n160 = call-poly "Enqueue Message.vi"("error in (no error)"=w616, "Message"="Sequence Start", "Message Queue"=w615) -> ("error out"=w614:errorcluster)  [unwired: 7 in, 1 out]
                          }
                          frame 9 {
                            # "Update Sonicator Setpoint"
                            n161 = Bundle By Name(cluster=T74 {"Auto?"=TRUE, "Manual Entry"=0.0, "Setpoint"=0.0}, "Auto?"=FALSE, "Manual Entry"=w638) -> (w636:T74)
                            n162 = Get Date/Time String() -> (time string=w627:string)  [unwired: 3 in, 1 out]
                            n163 = call-poly "Enqueue Message.vi"("error in (no error)"=w634, "Message Data"=w636, "Message"="Sequence Update", "Message Queue"=w635) -> ("error out"=w632:errorcluster, "dup Message Queue"=w631:refnum<queue>)  [unwired: 6 in]
                            n164 = Concatenate Strings("In Update Sonicator Setpoint" ("string"), "," ("string"), w627) -> (w626:string)
                            n165 = call-poly "Enqueue Message.vi"("error in (no error)"=w632, "Message"="Sequence Start", "Message Queue"=w631) -> ("error out"=w630:errorcluster)  [unwired: 7 in, 1 out]
                            n166 = call "Sequence Error Log.vi"("string"=w626, "Byte Stream File in"=w625) -> ()  [unwired: 10 in]
                          }
                          frame 2 {
                            # "DIO"
                            n167 = Bundle By Name(cluster=T74 {"Auto?"=TRUE, "Manual Entry"=0.0, "Setpoint"=0.0}, "Setpoint"=w653) -> (w650:T74)
                            n168 = Get Date/Time String() -> (time string=w643:string)  [unwired: 3 in, 1 out]
                            n169 = call-poly "Enqueue Message.vi"("error in (no error)"=w652, "Message Data"=w650, "Message"="Sequence Update", "Message Queue"=w651) -> ("error out"=w647:errorcluster, "dup Message Queue"=w648:refnum<queue>)  [unwired: 6 in]
                            n170 = Concatenate Strings("In DIO" ("string"), "," ("string"), w643) -> (w642:string)
                            n171 = call-poly "Enqueue Message.vi"("error in (no error)"=w647, "Message"="Sequence Start", "Message Queue"=w648) -> ("error out"=w646:errorcluster)  [unwired: 7 in, 1 out]
                            n172 = call "Sequence Error Log.vi"("string"=w642, "Byte Stream File in"=w641) -> ()  [unwired: 10 in]
                          }
                          frame 3, 4, 7, 8 {
                            # "Wait until"
                            n173 = Get Date/Time String() -> (time string=w658:string)  [unwired: 3 in, 1 out]
                            n174 = Concatenate Strings("In Wait Until" ("string"), "," ("string"), w658) -> (w657:string)
                            n175 = call "Sequence Error Log.vi"("string"=w657, "Byte Stream File in"=w656) -> ()  [unwired: 10 in]
                          }
                          frame Default {
                            n176 = Get Date/Time String() -> (time string=w664:string)  [unwired: 3 in, 1 out]
                            n177 = call-poly "Enqueue Message.vi"("error in (no error)"=w668, "Message"="Sequence Start", "Message Queue"=w669) -> ("error out"=w667:errorcluster)  [unwired: 7 in, 1 out]
                            n178 = Concatenate Strings("In Default" ("string"), "," ("string"), w664) -> (w663:string)
                            n179 = call "Sequence Error Log.vi"("string"=w663, "Byte Stream File in"=w662) -> ()  [unwired: 10 in]
                          }
                        }
                        n180 = Concatenate Strings("Queue Found" ("string"), "," ("string"), w551) -> (w550:string)
                        n181 = call "Sequence Error Log.vi"("string"=w550, "Byte Stream File in"=w549) -> ()  [unwired: 10 in]
                      }
                    }
                    n182 = call "Sequence Error Log.vi"("string"=w498, "Byte Stream File in"=w497) -> ()  [unwired: 10 in]
                    n183 = Get Date/Time In Seconds() -> (seconds since 1Jan1904=w509:timestamp)
                    n184 = call "Write to Log File.vi"("error in"=w507, "text"="Sequencer: Next Step") -> ()  [unwired: 9 in, 1 out]
                  }
                }
                n185 = Concatenate Strings("Not Done" ("string"), "," ("string"), w288) -> (w287:string)
                n186 = call "Sequence Error Log.vi"("string"=w287, "Byte Stream File in"=w286) -> ()  [unwired: 10 in]
              }
              frame True {
                w681 = TRUE
                # "This VI closes the Command Log File"
                # "Done"
                n187 = Get Date/Time String() -> (time string=w675:string)  [unwired: 3 in, 1 out]
                n188 = Wait (ms)(milliseconds to wait=u32 100) -> ()  [unwired: 1 out]
                n189 = Concatenate Strings("Done" ("string"), "," ("string"), w675) -> (w671:string)
                n190 = flat-sequence {
                  tunnel: w673 -> [w686]
                  tunnel: [w686] -> w672
                  tunnel: w671 -> [w687]
                  tunnel: [w689] -> w674
                  tunnel: w672 -> [w689]
                  tunnel: w674 -> [w690]
                  frame #0 {
                    n191 = call "Sequence Error Log.vi"("string"=w687, "Byte Stream File in"=w686) -> ()  [unwired: 10 in]
                  }
                  frame #1 {
                    n192 = Wait (ms)(milliseconds to wait=u32 3000) -> ()  [unwired: 1 out]
                  }
                  frame #2 {
                    n193 = Close File(refnum=w690) -> ()  [unwired: 1 in, 2 out]
                  }
                }
                n194 = call "Write to Log File.vi"("error in"=w679, "text"="Sequencer: Done") -> ()  [unwired: 9 in, 1 out]
                "Done" <- w681
              }
            }
            n195 = Get Date/Time String() -> (time string=w262:string)  [unwired: 3 in, 1 out]
            n196 = Concatenate Strings("Abort False" ("string"), "," ("string"), w262) -> (w261:string)
            n197 = call "Sequence Error Log.vi"("string"=w261, "Byte Stream File in"=w260) -> ()  [unwired: 10 in]
          }
          frame True {
            n198 = Get Date/Time String() -> (time string=w695:string)  [unwired: 3 in, 1 out]
            n199 = Concatenate Strings("Abort True" ("string"), "," ("string"), w695) -> (w692:string)
            n200 = flat-sequence {
              tunnel: [w705] -> _
              tunnel: [w705] -> w694
              tunnel: w692 -> [w706]
              tunnel: w691 -> [w705]
              tunnel: [w708] -> w693
              tunnel: w694 -> [w708]
              tunnel: w693 -> [w709]
              frame #0 {
                n201 = call "Sequence Error Log.vi"("string"=w706, "Byte Stream File in"=w705) -> ()  [unwired: 10 in]
              }
              frame #1 {
                n202 = Wait (ms)(milliseconds to wait=u32 3000) -> ()  [unwired: 1 out]
              }
              frame #2 {
                n203 = Close File(refnum=w709) -> ()  [unwired: 1 in, 2 out]
              }
            }
            n204 = Unbundle By Name(w701) -> ("Main Config.Steps"=w700:T57)
            n205 = Array Size(array=w700) -> (size(s)=w699:i32)
          }
        }
        n206 = call-poly "Enqueue Message.vi"("error in (no error)"=w246, "Message"="Run Sequence", "Message Queue"=w218) -> ("error out"=w245:errorcluster)  [unwired: 7 in, 1 out]
        n207 = control-ref of="This Application"() -> (w223:refnum<vi>)
        n208 = control-ref of="This VI"() -> (w221:refnum<vi>)
        n209 = property class="App"(reference=w223) -> ("App.AllVIs"=→"Application:All VIs In Memory":string[])  [unwired: 1 in, 2 out]
        n210 = property class="VI"(reference=w221) -> ("Metric.DataSize"=→"Metrics:Total Data Size":u32, "Metric.CodeSize"=→"Metrics:Code Size":u32)  [unwired: 1 in, 2 out]
      }
      frame "Exit" {
        n211 = call "Sequence Error Log.vi"("string"="In Exit", "Byte Stream File in"=w712) -> ()  [unwired: 10 in]
      }
    }
  }
  n212 = Release Queue(queue=w4) -> ()  [unwired: 2 in, 3 out]
  n213 = Merge Errors(w14, w12) -> (→"error out":errorcluster)
  n214 = Release Queue(queue=w3) -> ()  [unwired: 2 in, 3 out]
  n215 = Release Queue(queue=w2) -> ()  [unwired: 2 in, 3 out]
